vi "2024_06_02_sEQE.vi"() -> ()   [LabVIEW 2023]
uses:
  <vilib>/Utility/file.llb/Read From Spreadsheet File (DBL).vi
  <vilib>/gmath/NI_Gmath.lvlib
  <vilib>/Utility/file.llb/Write To Spreadsheet File (string).vi
  <vilib>/Utility/file.llb/Write To Spreadsheet File (DBL).vi
  Instrument Drivers/keithley_24xx/Keithley 24XX/Keithley 24XX.lvlib
  <vilib>/Analysis/NI_AALBase.lvlib
  E:/Old PC/desktop/Sensitive EQE Stuff/S-EQE (YJ)/Current Version/Thorlabs.MotionControl.Controls.dll
  <vilib>/Analysis/baseanly.llb/Mean (DBL).vi
  Files From Aram Lab/Labview VIs/EQE Newport/EQE Folder 2011/C/Program Files/National Instruments/LabVIEW 2017/instr.lib/Keithley 24XX/Public/Data/Read (Multiple Points).vi
  <vilib>/Analysis/1siggen.llb/Ramp Pattern by Samples.vi
  E:/Old PC/desktop/Sensitive EQE Stuff/S-EQE (YJ)/Current Version/Thorlabs.MotionControl.Benchtop.StepperMotorCLI.dll
panel:
  in  "Use Reference Detector":bool
  in  "Ref. Detector\nLockin Address":string="0:9"
  out "YJ@ AM1p5_1sun_photonflux_after interpolation":cluster{sgl[], "yi":dbl[]}(graph)
  out "70356_70316NS_473.txt":cluster{"all rows":dbl[], "all rows":dbl[]}(graph)={"all rows"=[0.0, 350.0, 355.0, 360.0, 365.0, 370.0, 375.0, 380.0, 385.0, 390.0, 395.0, 400.0, 405.0, 410.0, 415.0, 420.0, 425.0, 430.0, 435.0, 440.0, 445.0, 450.0, 455.0, 460.0, 465.0, 470.0, 475.0, 480.0, 485.0, 490.0, 495.0, 500.0, 505.0, 510.0, 515.0, 520.0, 525.0, 530.0, 535.0, 540.0, 545.0, 550.0, 555.0, 560.0, 565.0, 570.0, 575.0, 580.0, 585.0, 590.0, 595.0, 600.0, 605.0, 610.0, 615.0, 620.0, 625.0, 630.0, 635.0, 640.0, 645.0, 650.0, 655.0, 660.0, 665.0, 670.0, 675.0, 680.0, 685.0, 690.0, 695.0, 700.0, 705.0, 710.0, 715.0, 720.0, 725.0, 730.0, 735.0, 740.0, 745.0, 750.0, 755.0, 760.0, 765.0, 770.0, 775.0, 780.0, 785.0, 790.0, 795.0, 800.0, 805.0, 810.0, 815.0, 820.0, 825.0, 830.0, 835.0, 840.0, 845.0, 850.0, 855.0, 860.0, 865.0, 870.0, 875.0, 880.0, 885.0, 890.0, 895.0, 900.0, 905.0, 910.0, 915.0, 920.0, 925.0, 930.0, 935.0, 940.0, 945.0, 950.0, 955.0, 960.0, 965.0, 970.0, 975.0, 980.0, 985.0, 990.0, 995.0, 1000.0], "all rows"=[0.0, 0.000528, 0.000591, 0.00066, 0.000688, 0.000736, 0.000805, 0.000898, 0.000981, 0.001074, 0.001166, 0.001215, 0.001262, 0.001308, 0.001352, 0.001379, 0.001408, 0.001435, 0.001476, 0.001513, 0.00158, 0.001684, 0.001769, 0.001909, 0.002147, 0.002255, 0.002124, 0.002012, 0.001996, 0.001999, 0.00197, 0.001911, 0.001873, 0.001875, 0.00188, 0.001881, 0.001869, 0.001861, 0.001853, 0.00185, 0.001843, 0.001832, 0.001821, 0.001807, 0.001796, 0.001707, 0.001707, 0.001703, 0.001694, 0.001679, 0.00165, 0.001623, 0.001597, 0.001583, 0.001573, 0.001563, 0.00154, 0.001505, 0.001463, 0.00143, 0.001413, 0.001383, 0.001334, 0.001338, 0.001421, 0.001533, 0.001622, 0.00172, 0.00178, 0.001746, 0.001643, 0.001502, 0.001447, 0.001462, 0.001449, 0.001381, 0.001342, 0.001387, 0.001393, 0.001327, 0.001258, 0.001213, 0.001186, 0.001335, 0.001423, 0.001195, 0.000959, 0.000876, 0.000899, 0.000949, 0.00096, 0.000858, 0.000836, 0.000858, 0.001258, 0.002978, 0.00431, 0.003674, 0.002449, 0.001636, 0.001009, 0.000706, 0.000653, 0.000708, 0.000836, 0.001079, 0.001972, 0.003826, 0.004204, 0.003393, 0.003032, 0.00308, 0.002941, 0.002807, 0.003478, 0.003136, 0.001916, 0.001417, 0.001783, 0.002221, 0.002372, 0.002249, 0.001773, 0.001286, 0.001224, 0.001352, 0.002283, 0.002845, 0.002354, 0.002769, 0.002694, 0.001548]}
  out "YJ@ AM1p5_1sun_photonflux":cluster{"all rows":dbl[], "all rows":dbl[]}(graph)
  out "YJ@ KSC photodetector_Si_KSC.txt":cluster{"all rows":dbl[], "all rows":dbl[]}(graph)={"all rows"=[300.008, 319.964, 339.984, 359.993, 379.987, 399.968, 420.011, 440.038, 459.972, 479.966, 500.018, 519.975, 539.988, 559.982, 580.03, 599.981, 619.985, 639.966, 659.998, 680.005, 699.986, 720.017, 739.967, 759.964, 780.007, 800.019, 820.001, 840.026, 860.018, 879.977, 899.975, 920.013, 940.014, 959.979, 979.979, 1000.013, 1020.008, 1040.035, 1060.02, 1080.036, 1100.007, 1120.005, 1140.031, 1160.01, 1180.013, 1199.967, 1220.015, 1240.011, 1260.027, 1279.989, 1299.967, 1320.031, 1339.968, 1359.988, 1380.019, 1399.989, 1419.967, 1440.02, 1460.01, 1480.003, 1499.998, 1519.993, 1539.987, 1559.978, 1580.031, 1600.011, 1619.982, 1640.011, 1660.028, 1680.031, 1700.018, 1719.988, 1740.004, 1759.998, 1779.97, 1799.98], "all rows"=[22.44655, 29.69617, 32.2554, 33.72525, 44.35815, 59.92214, 69.4437, 73.3494, 73.77032, 72.54942, 69.11642, 66.67064, 64.65485, 63.26096, 62.09375, 61.11752, 61.04655, 61.202, 61.58933, 61.93196, 62.78305, 63.63964, 64.71529, 65.96744, 66.85927, 67.67915, 69.74085, 70.2863, 70.60146, 70.21348, 70.9341, 70.12613, 73.96691, 74.46643, 68.64919, 69.68867, 60.92799, 45.64385, 31.15813, 40.5953, 46.64548, 51.6218, 55.57125, 58.62437, 60.78791, 61.60885, 62.87273, 63.78579, 64.50757, 65.22985, 65.73163, 65.96526, 66.88447, 67.41929, 68.25897, 67.41081, 67.85151, 68.58292, 68.82948, 69.4892, 69.57728, 66.73863, 56.26826, 49.58999, 46.17923, 38.96613, 32.85697, 28.74497, 25.27677, 21.51941, 18.28548, 15.05667, 11.63632, 8.174946, 5.778172, 3.941114]}
  out "EQE data":dbl[](array[numeric])=[1.0630031270727235e-05, 2.224032414463779e-05, 3.860081064469949e-05, 5.693196442610228e-05, 7.885123421646286e-05, 0.00010409969342976093, 0.0001314805564755187, 0.00015761262171454783, 0.00018041038006170134, 0.0001994840969960363, 0.00021090229102895442, 0.00023735633466285739, 0.0002578215415721661, 0.00027707898011522546, 0.000293391194198478, 0.00031228191053828266, 0.0003277801105185816, 0.00033804597208761665, 0.0003483660325937561, 0.000366316440655734, 0.000385991499187727, 0.00042944053391323086, 0.000476573669238571, 0.0005114395273510304, 0.0005360105141446864, 0.0005518890213718105, 0.000554533572880275, 0.000545518555566591, 0.0005318038877618555, 0.0005248691938367492, 0.0005198235009739676, 0.0005139074960938296, 0.0005103600558364946, 0.0005099581034518405, 0.00051240772520516, 0.0005141352647575527, 0.0005160015247760515, 0.0005184268140636099, 0.0005215437161670573, 0.0005224495454948154, 0.0005239376083749391, 0.0005261934689407947, 0.0005275790524446975, 0.0005292676703269587, 3.684022279063007e-08, 3.001985497178216e-08, 3.011180213195135e-08, 6.376750400320879e-08, 6.389168834570928e-08, 6.305752891668185e-08]
  out "Applied Biases (V)":dbl[](array[numeric])
  out "Photonflux":dbl[](array[numeric])=[0.014905065, 0.017506614, 0.017369027, 0.018358634, 0.022533949, 0.017824447, 0.021478674, 0.020916015, 0.025070665, 0.025733941, 0.035944507, 0.037602476, 0.034673738, 0.041031376, 0.038050008, 0.042808518, 0.030334457, 0.043689466, 0.047907404, 0.05247181, 0.056603888, 0.05587127, 0.056733828, 0.057571786, 0.057155912, 0.062008993, 0.062646233, 0.061350661, 0.06412131, 0.065817672, 0.06231247, 0.06368507, 0.063682126, 0.06361276, 0.06390321, 0.066825496, 0.066029844, 0.06703682, 0.064570899, 0.067850258, 0.068313034, 0.069986046, 0.06657848, 0.069273794, 0.068116793, 0.068533433, 0.070266172, 0.07230634, 0.065238829, 0.068666398, 0.071397, 0.072684909, 0.0722573, 0.072904138, 0.073706888, 0.070706969, 0.070754315, 0.074050895, 0.074024843, 0.075784118, 0.071270366, 0.071316704, 0.074485562, 0.076240603, 0.076716567, 0.075993305, 0.076616551, 0.075958864, 0.065788756, 0.071271415, 0.072399581, 0.075140103, 0.075449669, 0.072589974, 0.057231812, 0.060699306, 0.066446604, 0.072195757, 0.072788353, 0.075094894, 0.074655186, 0.075408655, 0.016308308, 0.042329218, 0.072093563, 0.073580618, 0.073206001, 0.073358687, 0.069518471, 0.070099532, 0.06920471, 0.068468503, 0.06898524, 0.058849206, 0.057004485, 0.064503448, 0.061323463, 0.067565091, 0.068816583, 0.069280731, 0.061272947, 0.062962978, 0.068544733, 0.067204598, 0.067895507, 0.065414684, 0.066689918, 0.06740148, 0.066325028, 0.058730856, 0.053907082, 0.059644011, 0.045850113, 0.050064478, 0.055219293, 0.053054323, 0.032412728, 0.018917196, 0.035772012, 0.028065692, 0.011283836, 0.026279831, 0.032572479, 0.039208671, 0.049650887, 0.046388389, 0.047796935, 0.054673935, 0.058472923, 0.060332408, 0.059309566] format="%_6g"
  out "Gain (ohms, device)":dbl=1000.0
  out "Theta Device":dbl[](array[numeric])=[0.2700473581491309, 0.3151935612523878, 0.3840174824525091, 0.4343507017919065, 0.4985099952451927, 0.5521205217578055, 0.5932746185849422, 0.6229632673144792, 0.6603336996507065, 0.7021736365126859, 0.730245402674861, 0.7555351998358408, 0.7662251733370439, 0.7732410218978927, 0.7868403454893664, 0.8079871608349878, 0.833604606370508, 0.8512186270266459, 0.8571435014368394, 0.849056818576912, 0.8230805736611391, 0.797472299831973, 0.7949251497551506, 0.8229193465162005, 0.8544820820870439, 0.8945387107767107, 0.9101509858937846, 0.9180726508270242, 0.9138050297047764, 0.9170227233725305, 0.9185973975743922, 0.9127798480771039, 0.9020006840177286, 0.9085453202656186, 0.9004761874895579, 0.9060028541494218, 0.9048110423655178, 0.9040744374822528, 0.9048831165145835, 0.9054391223829343, 0.9038549251113345, 0.9099900965130696, 0.9091406237134004, 0.905658502401197, 0.9696722358529832, 0.9234869853808101, 0.8983673358190203, 0.6879877400938528, 0.6622097148496295, 0.6684745327767915]
  out "Calib Ref Current":dbl=1.455414177111583e-07
  out "Calib Photodet Current":dbl=1.1887647122469343e-06
  out "Calib detector EQE":dbl=0.7476
  out "Gain (ohms, ref)":dbl=1000.0
  out "Reference Current (A)":dbl[](array[numeric])=[0.001, 0.001, 0.001, 0.001, 0.001, 0.001, 0.001, 0.001, 0.001, 0.001, 0.001, 0.001, 0.001, 0.001, 0.001, 0.001, 0.001, 0.001, 0.001, 0.001, 0.001, 0.001, 0.001, 0.001, 0.001, 0.001, 0.001, 0.001, 0.001, 0.001, 0.001, 0.001, 0.001, 0.001, 0.001, 0.001, 0.001, 0.001, 0.001, 0.001, 0.001, 0.001, 0.001, 0.001, 0.001, 0.001, 0.001, 0.001, 0.001, 0.001]
  out "DC current (A)":dbl[](array[numeric])
  out "Device Current (A)":dbl[](array[numeric])=[3.506971664575117e-07, 7.419031190448685e-07, 1.3019656857999596e-06, 2.0716400561544406e-06, 3.0789055653533614e-06, 4.3415860564758075e-06, 5.833565646397709e-06, 7.606853812813335e-06, 9.409785273244745e-06, 1.1181556134893594e-05, 1.2640922706358269e-05, 1.4790296262148529e-05, 1.66779361860275e-05, 1.8581800630899686e-05, 2.037263692081463e-05, 2.1989850169184038e-05, 2.3400802905737088e-05, 2.4463332489649517e-05, 2.5549857791294584e-05, 2.6907472308324217e-05, 2.8393439889071035e-05, 3.1634879861557116e-05, 3.515617725054383e-05, 3.757203217284588e-05, 3.92134448854471e-05, 4.020658347574139e-05, 4.0227861162201044e-05, 3.9106902201208186e-05, 3.7668493858212035e-05, 3.6727997932696076e-05, 3.592994135283064e-05, 3.520567678187613e-05, 3.464992685110582e-05, 3.4310153885847094e-05, 3.416126068610294e-05, 3.4017503626001664e-05, 3.388111502655533e-05, 3.3779271471066726e-05, 3.3719894421586654e-05, 3.359634598967278e-05, 3.350940388445748e-05, 3.347026266189864e-05, 3.3374604444484423e-05, 3.3327354406248036e-05, 2.309060591324272e-09, 1.872836698407875e-09, 1.8698073076001774e-09, 3.944055898210585e-09, 3.936105226456829e-09, 3.869288620508274e-09]
  out "Wavelength range":sgl[](array[numeric])=[350.0, 355.0, 360.0, 365.0, 370.0, 375.0, 380.0, 385.0, 390.0, 395.0, 400.0, 405.0, 410.0, 415.0, 420.0, 425.0, 430.0, 435.0, 440.0, 445.0, 450.0, 455.0, 460.0, 465.0, 470.0, 475.0, 480.0, 485.0, 490.0, 495.0, 500.0, 505.0, 510.0, 515.0, 520.0, 525.0, 530.0, 535.0, 540.0, 545.0, 550.0, 555.0, 560.0, 565.0, 570.0, 575.0, 580.0, 585.0, 590.0, 595.0, 600.0, 605.0, 610.0, 615.0, 620.0, 625.0, 630.0, 635.0, 640.0, 645.0, 650.0, 655.0, 660.0, 665.0, 670.0, 675.0, 680.0, 685.0, 690.0, 695.0, 700.0, 705.0, 710.0, 715.0, 720.0, 725.0, 730.0, 735.0, 740.0, 745.0, 750.0, 755.0, 760.0, 765.0, 770.0, 775.0, 780.0, 785.0, 790.0, 795.0, 800.0, 805.0, 810.0, 815.0, 820.0, 825.0, 830.0, 835.0, 840.0, 845.0, 850.0, 855.0, 860.0, 865.0, 870.0, 875.0, 880.0, 885.0, 890.0, 895.0, 900.0, 905.0, 910.0, 915.0, 920.0, 925.0, 930.0, 935.0, 940.0, 945.0, 950.0, 955.0, 960.0, 965.0, 970.0, 975.0, 980.0, 985.0, 990.0, 995.0, 1000.0, 1005.0, 1010.0, 1015.0, 1020.0, 1025.0, 1030.0, 1035.0, 1040.0, 1045.0, 1050.0]
  in  "Tab Control":T1(tab)
  out "Auto Scale":string="Successful"
  out "Lockin status":bool
  out "Position of filter 1":dbl=360.0
  in  "Set as filter 1":bool
  out "Current degree":dbl=60.0
  out "Rotator status":bool
  in  "Anticlockwise":bool
  in  "clockwise":bool
  out "Mono status":bool
  out "Keithley status":bool
  in  "Initial devices":bool caption="To be initialized"
  in  "Start EXP":bool
  in  "Use Keithley for Bias?":bool
  in  "stop 3":bool caption="Be patient with this function"
  out "Current Wavelength":dbl=600.0 min=350.0 max=1100.0 step=1.0 format="%#.1f"
  out "Integrated Photocurrent (mA/cm2):":dbl format="%#_4f"
  in  "FileIO":enum32{"Take Calibration", "Take Measurement"}(tab)
  in  "Load Calibration Reference file":path=path "E:/Old PC/desktop/Sensitive EQE Stuff/S-EQE (YJ)/Calibration files (YJ)/JPJ New/KSC Combined Detector JPJ.txt"
  in  "70356_70316NS_473.txt":path=path "C:/Users/Admin/Desktop/Sensitive EQE Stuff/S-EQE (YJ)/Calibration files (YJ)/Si_Calibtation 19022019"
  out "70356_70316NS_473 File":cluster{sgl[], "yi":dbl[]}(graph)={[350.0, 355.0, 360.0, 365.0, 370.0, 375.0, 380.0, 385.0, 390.0, 395.0, 400.0, 405.0, 410.0, 415.0, 420.0, 425.0, 430.0, 435.0, 440.0, 445.0, 450.0, 455.0, 460.0, 465.0, 470.0, 475.0, 480.0, 485.0, 490.0, 495.0, 500.0, 505.0, 510.0, 515.0, 520.0, 525.0, 530.0, 535.0, 540.0, 545.0, 550.0, 555.0, 560.0, 565.0, 570.0, 575.0, 580.0, 585.0, 590.0, 595.0, 600.0, 605.0, 610.0, 615.0, 620.0, 625.0, 630.0, 635.0, 640.0, 645.0, 650.0, 655.0, 660.0, 665.0, 670.0, 675.0, 680.0, 685.0, 690.0, 695.0, 700.0, 705.0, 710.0, 715.0, 720.0, 725.0, 730.0, 735.0, 740.0, 745.0, 750.0, 755.0, 760.0, 765.0, 770.0, 775.0, 780.0, 785.0, 790.0, 795.0, 800.0, 805.0, 810.0, 815.0, 820.0, 825.0, 830.0, 835.0, 840.0, 845.0, 850.0, 855.0, 860.0, 865.0, 870.0, 875.0, 880.0, 885.0, 890.0, 895.0, 900.0, 905.0, 910.0, 915.0, 920.0, 925.0, 930.0, 935.0, 940.0, 945.0, 950.0, 955.0, 960.0, 965.0, 970.0, 975.0, 980.0, 985.0, 990.0, 995.0, 1000.0, 1005.0, 1010.0, 1015.0, 1020.0, 1025.0, 1030.0, 1035.0, 1040.0, 1045.0, 1050.0], "yi"=[32.991169783597385, 33.35846699985007, 33.728972631789546, 36.38799533860158, 39.04701804541362, 41.70604075222566, 44.368276213402716, 48.26297367599218, 52.15767113858164, 56.052368601171096, 59.937341812103966, 62.31262495335029, 64.68790809459661, 67.06319123584294, 69.43847437708925, 70.41666336445799, 71.39177196784341, 72.36688057122885, 73.34198917461427, 73.45417601284238, 73.55975442159125, 73.66533283034012, 73.76861022706812, 73.46329363208963, 73.15797703711112, 72.85266044213263, 72.54359903451027, 71.68757469778576, 70.83155036106125, 69.97552602433672, 69.11950168761221, 68.50586350553691, 67.89310106629253, 67.28033862704817, 66.66812189926549, 66.16450175236098, 65.66088160545645, 65.15726145855194, 64.65401341502451, 64.30543634190258, 63.95685926878063, 63.608282195658695, 63.259912026137265, 62.96880817537909, 62.677704324620905, 62.38660047386273, 62.095496623104545, 61.850561032028466, 61.60590412260037, 61.36124721317227, 61.1174525919816, 61.09971363977205, 61.081974687562486, 61.06423573535293, 61.046666698363445, 61.0855661528452, 61.12446560732696, 61.16336506180872, 61.20265740914537, 61.29933522464057, 61.39601304013578, 61.49269085563099, 61.58936425101214, 61.67499178137651, 61.76061931174089, 61.84624684210526, 61.931874372469636, 62.144721851258694, 62.357696677343476, 62.57067150342826, 62.783648685038195, 62.99746477010633, 63.21128085517448, 63.425096940242625, 63.63891302531077, 63.908309872180446, 64.17789633834586, 64.44748280451128, 64.71735635745361, 65.03044082012302, 65.34352528279241, 65.65660974546181, 65.96904185002245, 66.19152101980741, 66.41400018959237, 66.63647935937733, 66.8589585291623, 67.06383030581651, 67.26867739756146, 67.47352448930641, 67.67837158105138, 68.19307892102893, 68.70896822139926, 69.2248575217696, 69.74074682213993, 69.87701502122347, 70.01320728089887, 70.14939954057428, 70.28559180024969, 70.36471165666266, 70.4435331852741, 70.52235471388555, 70.601176242497, 70.50461565108473, 70.4074214028759, 70.31022715466707, 70.21430879587959, 70.39448181318133, 70.57465483048306, 70.75482784778478, 70.93309195278971, 70.73148251072962, 70.52987306866953, 70.32826362660944, 70.12665418454937, 71.08378061046947, 72.04392760311985, 73.0040745957702, 73.96422158842057, 74.09165864613072, 74.21675756924618, 74.34185649236163, 74.460321898, 73.00601189800001, 71.551701898, 70.09739189800001, 68.65027960167716, 68.90970857242688, 69.1691375431766, 69.42856651392633, 69.68799548467605, 67.50364818654668, 65.31293050712678, 63.12221282770695, 60.93149514828712, 57.11821185649378, 53.302328299296015, 49.48644474209825, 45.670561184900485, 42.04507092569435, 38.42092281461098]}
  out "Lamp Reference Photodetector Current":cluster{"Wavelength range":sgl[], dbl[]}(graph)={"Wavelength range"=[350.0, 355.0, 360.0, 365.0, 370.0, 375.0, 380.0, 385.0, 390.0, 395.0, 400.0, 405.0, 410.0, 415.0, 420.0, 425.0, 430.0, 435.0, 440.0, 445.0, 450.0, 455.0, 460.0, 465.0, 470.0, 475.0, 480.0, 485.0, 490.0, 495.0, 500.0, 505.0, 510.0, 515.0, 520.0, 525.0, 530.0, 535.0, 540.0, 545.0, 550.0, 555.0, 560.0, 565.0, 570.0, 575.0, 580.0, 585.0, 590.0, 595.0, 600.0, 605.0, 610.0, 615.0, 620.0, 625.0, 630.0, 635.0, 640.0, 645.0, 650.0, 655.0, 660.0, 665.0, 670.0, 675.0, 680.0, 685.0, 690.0, 695.0, 700.0, 705.0, 710.0, 715.0, 720.0, 725.0, 730.0, 735.0, 740.0, 745.0, 750.0, 755.0, 760.0, 765.0, 770.0, 775.0, 780.0, 785.0, 790.0, 795.0, 800.0, 805.0, 810.0, 815.0, 820.0, 825.0, 830.0, 835.0, 840.0, 845.0, 850.0, 855.0, 860.0, 865.0, 870.0, 875.0, 880.0, 885.0, 890.0, 895.0, 900.0, 905.0, 910.0, 915.0, 920.0, 925.0, 930.0, 935.0, 940.0, 945.0, 950.0, 955.0, 960.0, 965.0, 970.0, 975.0, 980.0, 985.0, 990.0, 995.0, 1000.0, 1005.0, 1010.0, 1015.0, 1020.0, 1025.0, 1030.0, 1035.0, 1040.0, 1045.0, 1050.0], [0.001, 0.001, 0.001, 0.001, 0.001, 0.001, 0.001, 0.001, 0.001, 0.001, 0.001, 0.001, 0.001, 0.001, 0.001, 0.001, 0.001, 0.001, 0.001, 0.001, 0.001, 0.001, 0.001, 0.001, 0.001, 0.001, 0.001, 0.001, 0.001, 0.001, 0.001, 0.001, 0.001, 0.001, 0.001, 0.001, 0.001, 0.001, 0.001, 0.001, 0.001, 0.001, 0.001, 0.001, 0.001, 0.001, 0.001, 0.001, 0.001, 0.001]}
  out "Device Current":cluster{"Wavelength range":sgl[], dbl[]}(graph)={"Wavelength range"=[350.0, 355.0, 360.0, 365.0, 370.0, 375.0, 380.0, 385.0, 390.0, 395.0, 400.0, 405.0, 410.0, 415.0, 420.0, 425.0, 430.0, 435.0, 440.0, 445.0, 450.0, 455.0, 460.0, 465.0, 470.0, 475.0, 480.0, 485.0, 490.0, 495.0, 500.0, 505.0, 510.0, 515.0, 520.0, 525.0, 530.0, 535.0, 540.0, 545.0, 550.0, 555.0, 560.0, 565.0, 570.0, 575.0, 580.0, 585.0, 590.0, 595.0, 600.0, 605.0, 610.0, 615.0, 620.0, 625.0, 630.0, 635.0, 640.0, 645.0, 650.0, 655.0, 660.0, 665.0, 670.0, 675.0, 680.0, 685.0, 690.0, 695.0, 700.0, 705.0, 710.0, 715.0, 720.0, 725.0, 730.0, 735.0, 740.0, 745.0, 750.0, 755.0, 760.0, 765.0, 770.0, 775.0, 780.0, 785.0, 790.0, 795.0, 800.0, 805.0, 810.0, 815.0, 820.0, 825.0, 830.0, 835.0, 840.0, 845.0, 850.0, 855.0, 860.0, 865.0, 870.0, 875.0, 880.0, 885.0, 890.0, 895.0, 900.0, 905.0, 910.0, 915.0, 920.0, 925.0, 930.0, 935.0, 940.0, 945.0, 950.0, 955.0, 960.0, 965.0, 970.0, 975.0, 980.0, 985.0, 990.0, 995.0, 1000.0, 1005.0, 1010.0, 1015.0, 1020.0, 1025.0, 1030.0, 1035.0, 1040.0, 1045.0, 1050.0], [3.506971664575117e-07, 7.419031190448685e-07, 1.3019656857999596e-06, 2.0716400561544406e-06, 3.0789055653533614e-06, 4.3415860564758075e-06, 5.833565646397709e-06, 7.606853812813335e-06, 9.409785273244745e-06, 1.1181556134893594e-05, 1.2640922706358269e-05, 1.4790296262148529e-05, 1.66779361860275e-05, 1.8581800630899686e-05, 2.037263692081463e-05, 2.1989850169184038e-05, 2.3400802905737088e-05, 2.4463332489649517e-05, 2.5549857791294584e-05, 2.6907472308324217e-05, 2.8393439889071035e-05, 3.1634879861557116e-05, 3.515617725054383e-05, 3.757203217284588e-05, 3.92134448854471e-05, 4.020658347574139e-05, 4.0227861162201044e-05, 3.9106902201208186e-05, 3.7668493858212035e-05, 3.6727997932696076e-05, 3.592994135283064e-05, 3.520567678187613e-05, 3.464992685110582e-05, 3.4310153885847094e-05, 3.416126068610294e-05, 3.4017503626001664e-05, 3.388111502655533e-05, 3.3779271471066726e-05, 3.3719894421586654e-05, 3.359634598967278e-05, 3.350940388445748e-05, 3.347026266189864e-05, 3.3374604444484423e-05, 3.3327354406248036e-05, 2.309060591324272e-09, 1.872836698407875e-09, 1.8698073076001774e-09, 3.944055898210585e-09, 3.936105226456829e-09, 3.869288620508274e-09]}
  in  "Step size (nm)":sgl=5.0 min=1 step=0.1
  in  "End Wavelength (nm)":sgl=1050.0 min=250 max=1350 step=0.1
  in  "Start Wavelength (nm)":sgl=350.0 min=250 max=1200 step=0.1
  in  "Bias (V)":dbl min=-30.0 max=10.0
  out "EQE":cluster{"Wavelength range":sgl[], dbl[]}(graph)={"Wavelength range"=[350.0, 355.0, 360.0, 365.0, 370.0, 375.0, 380.0, 385.0, 390.0, 395.0, 400.0, 405.0, 410.0, 415.0, 420.0, 425.0, 430.0, 435.0, 440.0, 445.0, 450.0, 455.0, 460.0, 465.0, 470.0, 475.0, 480.0, 485.0, 490.0, 495.0, 500.0, 505.0, 510.0, 515.0, 520.0, 525.0, 530.0, 535.0, 540.0, 545.0, 550.0, 555.0, 560.0, 565.0, 570.0, 575.0, 580.0, 585.0, 590.0, 595.0, 600.0, 605.0, 610.0, 615.0, 620.0, 625.0, 630.0, 635.0, 640.0, 645.0, 650.0, 655.0, 660.0, 665.0, 670.0, 675.0, 680.0, 685.0, 690.0, 695.0, 700.0, 705.0, 710.0, 715.0, 720.0, 725.0, 730.0, 735.0, 740.0, 745.0, 750.0, 755.0, 760.0, 765.0, 770.0, 775.0, 780.0, 785.0, 790.0, 795.0, 800.0, 805.0, 810.0, 815.0, 820.0, 825.0, 830.0, 835.0, 840.0, 845.0, 850.0, 855.0, 860.0, 865.0, 870.0, 875.0, 880.0, 885.0, 890.0, 895.0, 900.0, 905.0, 910.0, 915.0, 920.0, 925.0, 930.0, 935.0, 940.0, 945.0, 950.0, 955.0, 960.0, 965.0, 970.0, 975.0, 980.0, 985.0, 990.0, 995.0, 1000.0, 1005.0, 1010.0, 1015.0, 1020.0, 1025.0, 1030.0, 1035.0, 1040.0, 1045.0, 1050.0], [1.0630031270727235e-05, 2.224032414463779e-05, 3.860081064469949e-05, 5.693196442610228e-05, 7.885123421646286e-05, 0.00010409969342976093, 0.0001314805564755187, 0.00015761262171454783, 0.00018041038006170134, 0.0001994840969960363, 0.00021090229102895442, 0.00023735633466285739, 0.0002578215415721661, 0.00027707898011522546, 0.000293391194198478, 0.00031228191053828266, 0.0003277801105185816, 0.00033804597208761665, 0.0003483660325937561, 0.000366316440655734, 0.000385991499187727, 0.00042944053391323086, 0.000476573669238571, 0.0005114395273510304, 0.0005360105141446864, 0.0005518890213718105, 0.000554533572880275, 0.000545518555566591, 0.0005318038877618555, 0.0005248691938367492, 0.0005198235009739676, 0.0005139074960938296, 0.0005103600558364946, 0.0005099581034518405, 0.00051240772520516, 0.0005141352647575527, 0.0005160015247760515, 0.0005184268140636099, 0.0005215437161670573, 0.0005224495454948154, 0.0005239376083749391, 0.0005261934689407947, 0.0005275790524446975, 0.0005292676703269587, 3.684022279063007e-08, 3.001985497178216e-08, 3.011180213195135e-08, 6.376750400320879e-08, 6.389168834570928e-08, 6.305752891668185e-08]}
  out "EQE (log scale)":cluster{"Wavelength range":sgl[], dbl[]}(graph)={"Wavelength range"=[350.0, 355.0, 360.0, 365.0, 370.0, 375.0, 380.0, 385.0, 390.0, 395.0, 400.0, 405.0, 410.0, 415.0, 420.0, 425.0, 430.0, 435.0, 440.0, 445.0, 450.0, 455.0, 460.0, 465.0, 470.0, 475.0, 480.0, 485.0, 490.0, 495.0, 500.0, 505.0, 510.0, 515.0, 520.0, 525.0, 530.0, 535.0, 540.0, 545.0, 550.0, 555.0, 560.0, 565.0, 570.0, 575.0, 580.0, 585.0, 590.0, 595.0, 600.0, 605.0, 610.0, 615.0, 620.0, 625.0, 630.0, 635.0, 640.0, 645.0, 650.0, 655.0, 660.0, 665.0, 670.0, 675.0, 680.0, 685.0, 690.0, 695.0, 700.0, 705.0, 710.0, 715.0, 720.0, 725.0, 730.0, 735.0, 740.0, 745.0, 750.0, 755.0, 760.0, 765.0, 770.0, 775.0, 780.0, 785.0, 790.0, 795.0, 800.0, 805.0, 810.0, 815.0, 820.0, 825.0, 830.0, 835.0, 840.0, 845.0, 850.0, 855.0, 860.0, 865.0, 870.0, 875.0, 880.0, 885.0, 890.0, 895.0, 900.0, 905.0, 910.0, 915.0, 920.0, 925.0, 930.0, 935.0, 940.0, 945.0, 950.0, 955.0, 960.0, 965.0, 970.0, 975.0, 980.0, 985.0, 990.0, 995.0, 1000.0, 1005.0, 1010.0, 1015.0, 1020.0, 1025.0, 1030.0, 1035.0, 1040.0, 1045.0, 1050.0], [1.0630031270727235e-05, 2.224032414463779e-05, 3.860081064469949e-05, 5.693196442610228e-05, 7.885123421646286e-05, 0.00010409969342976093, 0.0001314805564755187, 0.00015761262171454783, 0.00018041038006170134, 0.0001994840969960363, 0.00021090229102895442, 0.00023735633466285739, 0.0002578215415721661, 0.00027707898011522546, 0.000293391194198478, 0.00031228191053828266, 0.0003277801105185816, 0.00033804597208761665, 0.0003483660325937561, 0.000366316440655734, 0.000385991499187727, 0.00042944053391323086, 0.000476573669238571, 0.0005114395273510304, 0.0005360105141446864, 0.0005518890213718105, 0.000554533572880275, 0.000545518555566591, 0.0005318038877618555, 0.0005248691938367492, 0.0005198235009739676, 0.0005139074960938296, 0.0005103600558364946, 0.0005099581034518405, 0.00051240772520516, 0.0005141352647575527, 0.0005160015247760515, 0.0005184268140636099, 0.0005215437161670573, 0.0005224495454948154, 0.0005239376083749391, 0.0005261934689407947, 0.0005275790524446975, 0.0005292676703269587, 3.684022279063007e-08, 3.001985497178216e-08, 3.011180213195135e-08, 6.376750400320879e-08, 6.389168834570928e-08, 6.305752891668185e-08]}
  in  "Pause Request":bool
  out "Paused":bool
  in  "Keithley 2400 address":refnum<visa-resource-name>="GPIB0::24::INSTR"
  in  "AM1p5_1sun_photoflux":path=path "E:/Old PC/desktop/Sensitive EQE Stuff/S-EQE (YJ)/Calibration files (YJ)/AM1p5_1sun_photonflux.xls"
  in  "Step":string(combo)="60"
  out "Delay (s)":sgl=1.5 format="%#.2f"
  in  "lockin":T2={"Lock-in VISA address"="GPIB0::8::INSTR", "Integration (ms) "=3000, "data storage rate (Hz)"=enum."16"}
  out "GPIB address":string="0:8"
  in  "Autogain":bool
  in  "stop":bool
  out "Current Filter":dbl=5.0
  in  "Autoscale Starts":dbl=350.0
  in  "Auto Gain Point Separation":i32=1
  in  "Average Method":bool=TRUE
  in  "Delay-2 (s)":dbl=5.0
  in  "MC Config File (19523)":path=path "E:/Old PC/desktop/MSH-300/MSH-300/Configurations/config/19523/LOT_MSH-300_SN19523 new (1).xml"
  out "Current wavelength test (nm)":dbl=550.0 format="%#.1f"
  in  "Goto wavelength":bool
  in  "Wavelength (nm)":sgl=550.0 min=250 max=1350 step=0.1 format="%.1f"
  in  "Skip reset after\nmeasurement":bool
  in  "Save File (Prompt if blank)":path
  in  "Voltage Profile":path=path "C:/Labview VIs/Voltage Profiles/ETH_1.xls"
  in  "Load Voltage Profile?":bool
  in  "Lock-In IV curve calb tab":enum32{"Calibrate", "Scan"}(tab)
  in  "Load Calibration Reference file":path=path "C:/Labview VIs/Photodiode Calibration Files/70356_70316NS_473.txt"
  in  "Calibration Value":dbl=11.66 min=0.0
  in  "Use Reference Detector?":bool=TRUE
  in  "Lockin Parameters":T3={"Device Lockin Address"="1:8", "Ref. Lockin Address"="1:9", "Wait (ms)"=500.0, "Integration (ms) "=2000, "data storage rate (Hz)"=enum."32"}
  in  "Monochromator Controls":T4={"Wavelength (nm)"=550.0, "Shutter"=enum."Open"} {"Wavelength (nm)" min=0 max=1400 step=0.1}
  out "EQE(V)":cluster{dbl[], dbl[]}(graph)={[0.0], [5.834199398071779]}
  out "Reference Lockin Current":cluster{"Wavelengths":dbl[], dbl[]}(graph)={"Wavelengths"=[0.0], [1.455414177111583e-07]}
  out "Device Lockin Current":cluster{dbl[], dbl[]}(graph)={[0.0], [1.1887647122469343e-06]}
  out "Device DC current":cluster{dbl[], dbl[]}(graph)={[0.0], [1.0150755315407879e-06]}
  in  "Bias Parameters":T5={"VISA resource name"="GPIB0::24::INSTR", "Start Bias (V)"=1.0, "End Bias (V) "=-10.0, "Number of points minus 1"=50, "Compliance (A)"=0.05} {"Number of points minus 1" min=0}
  in  "stop 2":bool
  in  "BenchtopStepperControl":refnum<k24>(container)
  out "BenchtopStepperMotor":refnum<k24>
  # "YJ@Select the measurement rage"
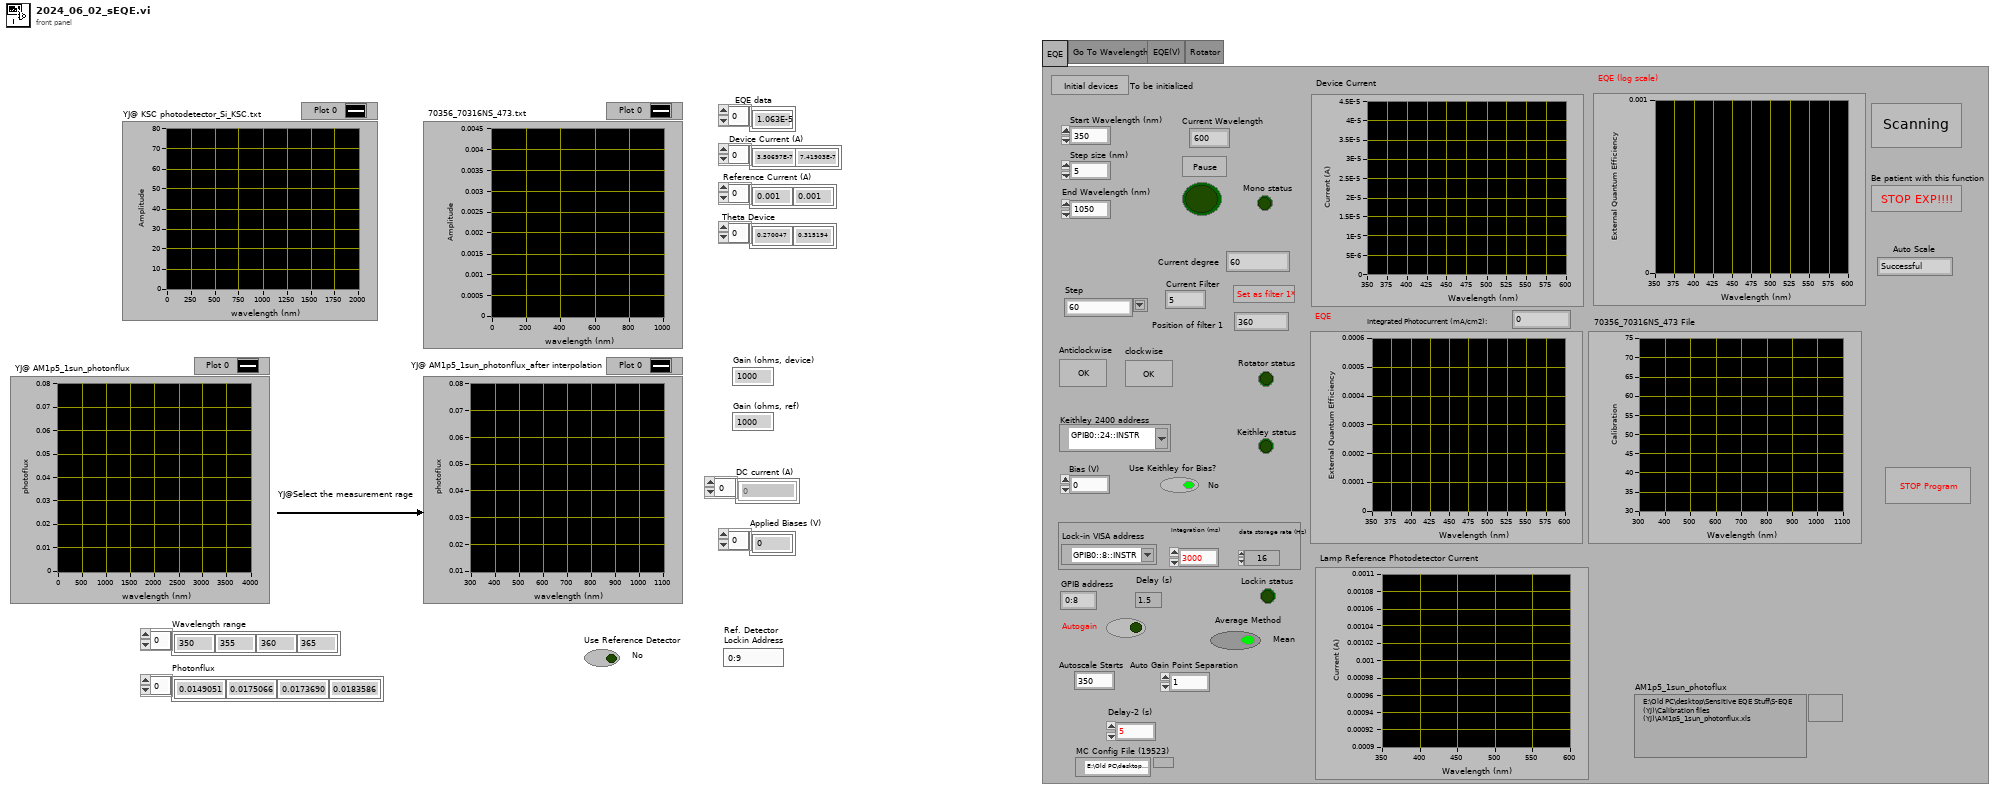
[diagram p1: front panel]
types:
  T1 = enum32{"EQE", "Go To Wavelength", "EQE(V)", "Rotator"}
  T2 = cluster{"Lock-in VISA address":refnum<visa-resource-name>, "Integration (ms) ":u32, "data storage rate (Hz)":enum16{".0625", ".125", ".25", ".5", "1", "2", "4", "8", "16", "32", "64", "128", "256", "512"}}
  T3 = cluster{"Device Lockin Address":string, "Ref. Lockin Address":string, "Wait (ms)":dbl, "Integration (ms) ":u32, "data storage rate (Hz)":enum16{".0625", ".125", ".25", ".5", "1", "2", "4", "8", "16", "32", "64", "128", "256", "512"}}
  T4 = cluster{"Wavelength (nm)":sgl, "Shutter":enum16{"Open", "Closed"}}
  T5 = cluster{"VISA resource name":refnum<visa-resource-name>, "Start Bias (V)":dbl, "End Bias (V) ":dbl, "Number of points minus 1":i16, "Compliance (A)":dbl}
  T6 = enum8{"Enabled", "Disabled", "Disabled and Grayed Out"}
  T7 = enum16{".0625", ".125", ".25", ".5", "1", "2", "4", "8", "16", "32", "64", "128", "256", "512"}
  T8 = cluster{"error":bool, "code":i32, "source":string}
  T9 = cluster{"Applied Biases (V)":dbl[], "DC current (A)":dbl[]}
  T10 = cluster{"Applied Biases (V)":dbl[], "Device Current (A)":dbl[]}
  T11 = cluster{"Applied Biases (V)":dbl[], "Reference Current (A)":dbl[]}
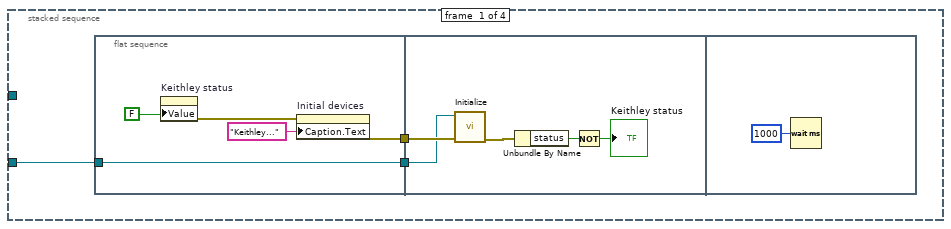
[diagram p6: hidden frame]
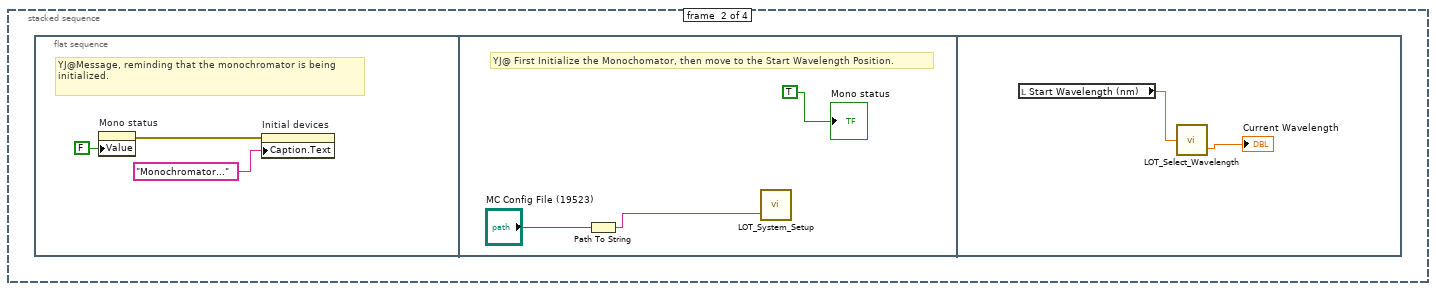
[diagram p7: hidden frame]
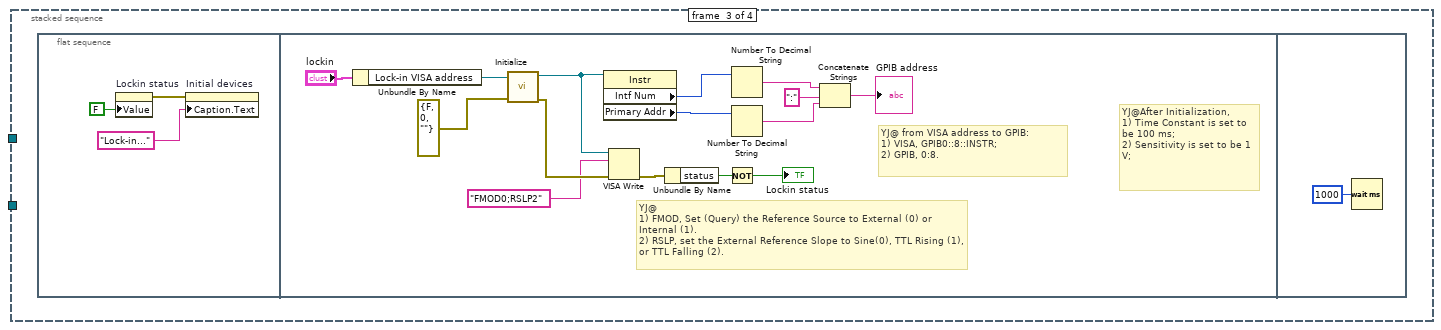
[diagram p8: hidden frame]
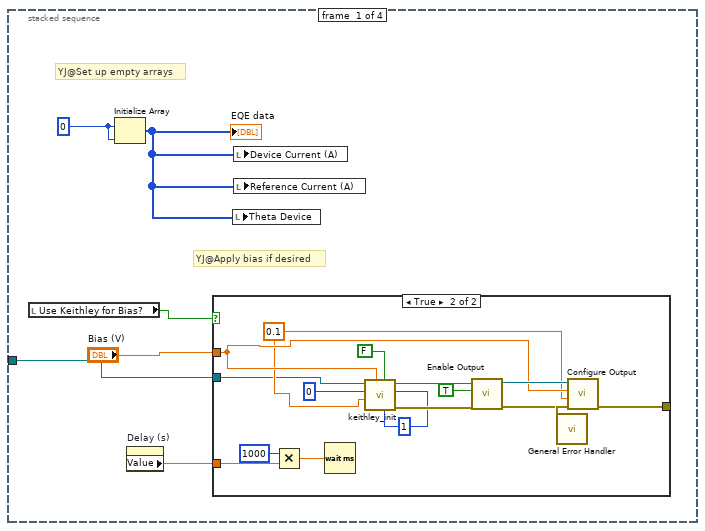
[diagram p10: hidden frame]
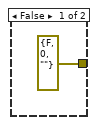
[diagram p11: hidden frame]
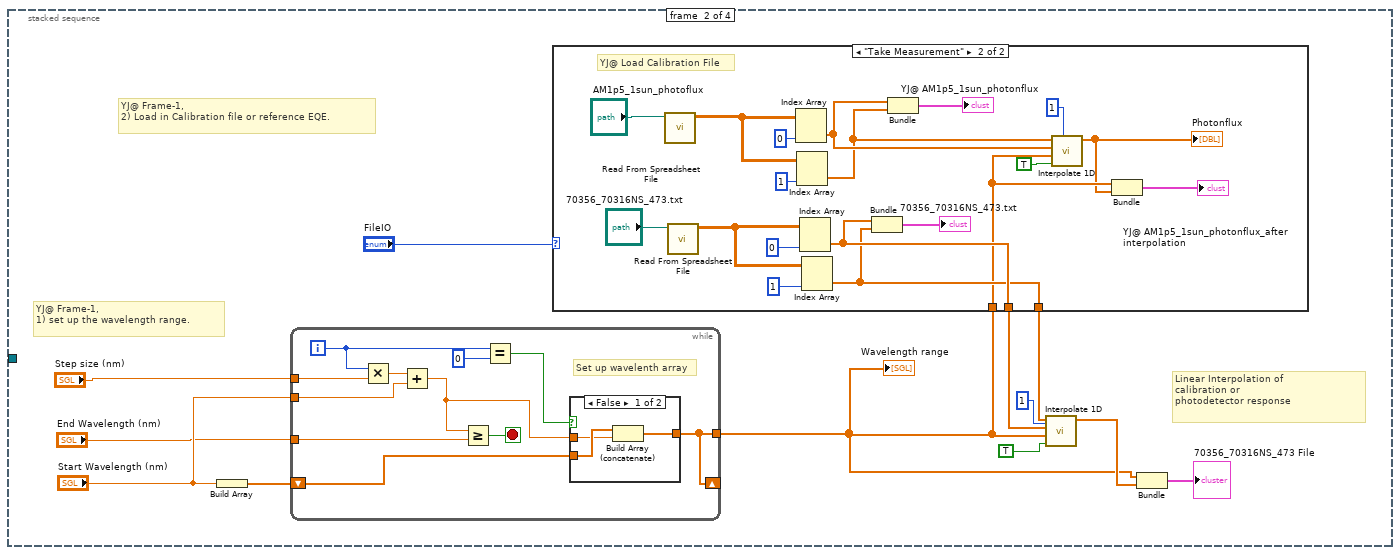
[diagram p12: hidden frame]
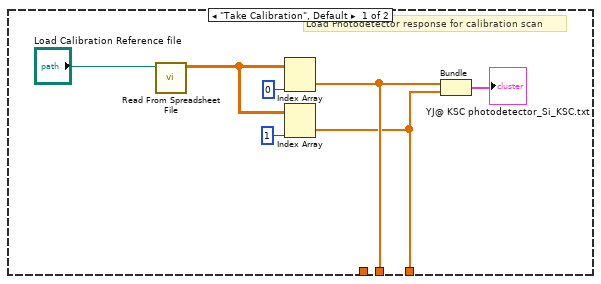
[diagram p14: hidden frame]
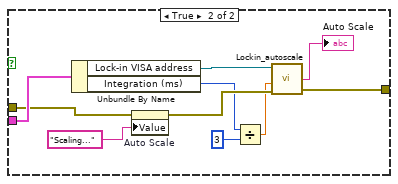
[diagram p15: hidden frame]
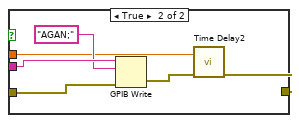
[diagram p17: hidden frame]
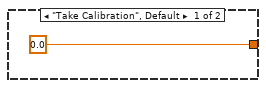
[diagram p18: hidden frame]
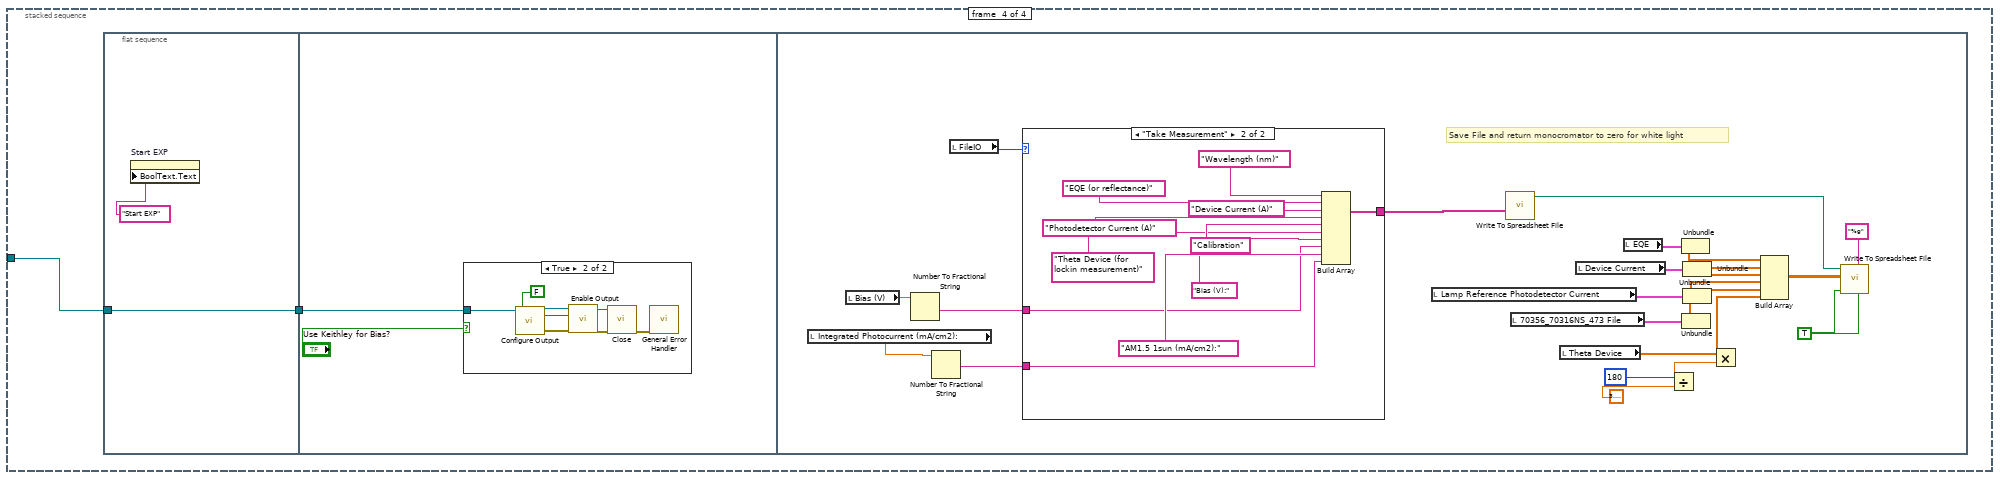
[diagram p19: hidden frame]
diagram:
  w2 = FALSE ("Lockin status")
  # "YJ@\n1)Delay time is one half of the integration;\n2)Be careful for the unit conversion, Integration being ms, and delay being second."
  n1 = property on="Rotator status" class="Bool (strict)"("Value"=w2) -> ()  [unwired: 2 in, 2 out]
  n2 = property on="Mono status" class="Bool (strict)"("Value"=w2) -> ()  [unwired: 2 in, 2 out]
  n3 = property on="Keithley status" class="Bool (strict)"("Value"=w2) -> ()  [unwired: 2 in, 2 out]
  n4 = property on="Lockin status" class="Bool (strict)"("Value"=w2) -> (error out=w3:errorcluster)  [unwired: 2 in, 1 out]
  n5 = property on="Position of filter 1" class="DigNum (strict)"("Value"=360.0 ("Position of filter 1")) -> ()  [unwired: 2 in, 2 out]
  n6 = property on="Start EXP" class="Bool"(error in=w3, "BoolText.Text"="Start EXP" ("Boolean Text.Text")) -> (error out=w5:errorcluster)  [unwired: 1 in, 1 out]
  n7 = property on="Initial devices" class="Bool"(error in=w5, "Caption.Text"="To be initialized") -> (error out=w6:errorcluster)  [unwired: 1 in, 1 out]
  n8 = while "Level-1, while loop, controlling the whole S-EQE program." {
    tunnel: w6 -> [w8]
    stop <- "stop" stop-if-true
    # "YJ@four tabs:\n1, EQE;\n2, Go To Wavelength;\n3, EQE (V);\n4, Rotator;"
    n9 = property on="lockin" class="Clust (strict)"(error in=w8) -> ("Value"=w10:T2)  [unwired: 1 in, 2 out]
    n10 = Unbundle By Name(w10) -> ("Integration (ms)"=w11:u32)
    n11 = Wait (ms)(milliseconds to wait=u32 20) -> ()  [unwired: 1 out]
    n12 = Divide(x=w11, y=u32 2000) -> (x/y=→"Delay (s)":dbl)
    n13 = case "Level-2, case structure, controlled by Tab Control, choosing specific pages." shown="\"EQE\", Default" "Tab Control" {
      tunnel: "Keithley 2400 address" -> [w31 _ _]
      frame "EQE", Default {
        n14 = case "Level-3, case structure, controlled by OK buttong, determine whether to initiate the units or not." shown="True" "Initial devices" {
          tunnel: w31 -> [_ w55]
          tunnel: "BenchtopStepperControl" -> [_ w54]
          frame False {
          }
          frame True {
            # "YJ@A sequence of Initialization:\nFrame-0, Keithley;\nFrame-1,Mono-chromator;\nFrame-2, Lock-in;\nFrame-3, Rotator."
            n15 = stacked-sequence "Level-4, flat sequence structure, inside the case structure, starts a sequence of unit initialization." {
              tunnel: w55 -> [w56 _ _ _]
              tunnel: w54 -> [_ _ _ w111]
              frame #0 {
                n16 = flat-sequence {
                  tunnel: [w60] -> w58
                  tunnel: [w59] -> w57
                  tunnel: w56 -> [w59]
                  tunnel: w58 -> [w66]
                  tunnel: w57 -> [w64]
                  frame #0 {
                    n17 = property on="Keithley status" class="Bool (strict)"("Value"=FALSE ("Keithley status")) -> (error out=w62:errorcluster)  [unwired: 2 in, 1 out]
                    n18 = property on="Initial devices" class="Bool"(error in=w62, "Caption.Text"="Keithley...") -> (error out=w60:errorcluster)  [unwired: 1 in, 1 out]
                  }
                  frame #1 {
                    n19 = call "Initialize.vi"("error in (no error)"=w66, "VISA resource name"=w64) -> ("error out"=w65:errorcluster)  [unwired: 8 in, 1 out]
                    n20 = Unbundle By Name(w65) -> ("status"=w68:bool)
                    n21 = Not(x=w68) -> (.not. x?=→"Keithley status":bool)
                  }
                  frame #2 {
                    n22 = Wait (ms)(milliseconds to wait=u32 1000) -> ()  [unwired: 1 out]
                  }
                }
              }
              frame #1 {
                n23 = flat-sequence {
                  frame #0 {
                    # "YJ@Message, reminding that the monochromator is being initialized."
                    n24 = property on="Mono status" class="Bool (strict)"("Value"=FALSE ("Mono status")) -> (error out=w70:errorcluster)  [unwired: 2 in, 1 out]
                    n25 = property on="Initial devices" class="Bool"(error in=w70, "Caption.Text"="Monochromator...") -> ()  [unwired: 1 in, 2 out]
                  }
                  frame #1 {
                    # "YJ@ First Initialize the Monochomator, then move to the Start Wavelength Position."
                    n26 = Path To String(path="MC Config File (19523)") -> (string=w74:string)
                    n27 = call "LOT_System_Setup.vi"("CFG File Path"=w74) -> ()  [unwired: 2 in, 1 out]
                    "Mono status" <- TRUE
                  }
                  frame #2 {
                    n28 = local read "Start Wavelength (nm)"() -> (w77:sgl)
                    n29 = call "LOT_Select_Wavelength.vi"("Input Wavelength"=w77) -> ("Current Wavelength"=→"Current Wavelength":dbl)  [unwired: 1 out]
                  }
                }
              }
              frame #2 {
                n30 = flat-sequence {
                  frame #0 {
                    n31 = property on="Lockin status" class="Bool (strict)"("Value"=FALSE ("Mono status")) -> (error out=w78:errorcluster)  [unwired: 2 in, 1 out]
                    n32 = property on="Initial devices" class="Bool"(error in=w78, "Caption.Text"="Lock-in...") -> ()  [unwired: 1 in, 2 out]
                  }
                  frame #1 {
                    # "YJ@After Initialization, \n1) Time Constant is set to be 100 ms;\n2) Sensitivity is set to be 1 V;"
                    # "YJ@ \n1) FMOD, Set (Query) the Reference Source to External (0) or Internal (1).\n2) RSLP, set the External Reference Slope to Sine(0), TTL Rising (1), or TTL Falling (2)."
                    # "YJ@ from VISA address to GPIB:\n1) VISA, GPIB0::8::INSTR;\n2) GPIB, 0:8."
                    n33 = Unbundle By Name("lockin") -> ("Lock-in VISA address"=w92:refnum<visa-resource-name>)
                    n34 = call "Initialize.vi"("error in (no error)"=errorcluster {"status"=FALSE, "code"=0, "source"=""}, "VISA resource name"=w92) -> ("error out"=w85:errorcluster, "VISA resource name out"=w82:refnum<visa-resource-name>)  [unwired: 8 in]
                    n35 = property class="Instr"(reference=w82) -> ("Intf Num"=w91:u16, "Primary Addr"=w87:u16)  [unwired: 1 in, 2 out]
                    n36 = VISA Write(VISA resource name=w82, write buffer="FMOD0;RSLP2", error in (no error)=w85) -> (error out=w81:errorcluster)  [unwired: 2 out]
                    n37 = Unbundle By Name(w81) -> ("status"=w94:bool)
                    n38 = Not(x=w94) -> (.not. x?=→"Lockin status":bool)
                    n39 = Number To Decimal String(number=w91) -> (decimal integer string=w89:string)  [unwired: 1 in]
                    n40 = Number To Decimal String(number=w87) -> (decimal integer string=w86:string)  [unwired: 1 in]
                    n41 = Concatenate Strings(w89, ":" ("string"), w86) -> (→"GPIB address":string)
                  }
                  frame #2 {
                    n42 = Wait (ms)(milliseconds to wait=u32 1000) -> ()  [unwired: 1 out]
                  }
                }
              }
              frame #3 {
                # "YJ@Ignor the rever and forward limit switch, so the rotator can move in both directions."
                # "YJ@ \n1, No Error, True, Execute;\n0, Error, False;"
                # "YJ@ Avoid endless Initialization.\n1) Include the Initialization Process in the case structure."
                # "YJ@This APT homing subVI only execute when the motor is not at home."
                # "YJ@this output is always zero."
                # "YJ@Motor homed (1 - homed, 0 - not homed)."
                # "YJ@LED is light if there is No Error AND Motor Moved Home."
                # "YJ@ After no:\n0 for Error;\n1 for No Error;"
                # "YJ@ Frame-3, Initialize Rotator."
                n43 = property on="Rotator status" class="Bool (strict)"(error in=errorcluster {"status"=FALSE, "code"=0, "source"=""} ("error in (no error)"), "Value"=FALSE ("x .and. y?")) -> (error out=w115:errorcluster)  [unwired: 1 in, 1 out]
                n44 = property on="Initial devices" class="Bool"(error in=w115, "Caption.Text"="Rotator...") -> (error out=w97:errorcluster)  [unwired: 1 in, 1 out]
                n45 = property class="BenchtopStepperControl"(reference=w111, error in=w97, "SerialNumber"="40846753") -> (reference out=w109:refnum<k24>)  [unwired: 1 out]
                n46 = invoke class="BenchtopStepperControl" method="CreateDevice"(reference=w109) -> (reference out=w108:refnum<k24>)  [unwired: 2 in, 2 out]
                n47 = property class="BenchtopStepperControl"(reference=w108) -> (error out=w106:errorcluster, "BenchtopStepperMotor"=w107:refnum<k24>)  [unwired: 1 in, 1 out]
                "BenchtopStepperMotor" <- w107
                n48 = call "Kinesis Home.vi"("error in (no error)"=w106, ".NET Refnum in"=w107) -> ("error out"=w104:errorcluster, ".NET Refnum out"=w105:refnum<k24>)  [unwired: 8 in]
                n49 = call "Kinesis Move.vi"("error in (no error)"=w104, "Move Position"=0.0, ".NET Refnum in"=w105) -> ("error out"=w101:errorcluster, "Position"=→"Current degree":dbl)  [unwired: 7 in]
                n50 = Unbundle By Name(w101) -> ("status"=w100:bool)
                n51 = Not(x=w100) -> (.not. x?=→"Rotator status":bool)
                n52 = property on="Position of filter 1" class="DigNum (strict)"() -> ("Value"=w112:dbl)  [unwired: 2 in, 2 out]
                n53 = Divide(x=w112, y=360.0) -> ()  [unwired: 1 out]
                n54 = property on="Initial devices" class="Bool"(error in=w101, "Caption.Text"="Initialization completed") -> ()  [unwired: 1 in, 2 out]
              }
            }
          }
        }
        n55 = case "Level-3, case structure, controlled by an OK buttong, determine whether to Anticlosewisely rotate the rotator." shown="True" "Anticlockwise" {
          frame False {
          }
          frame True {
            n56 = property on="Current degree" class="DigNum (strict)"() -> ("Value"=w51:dbl)  [unwired: 2 in, 2 out]
            n57 = local read "BenchtopStepperMotor"() -> (w47:refnum<k24>)
            n58 = Fract/Exp String To Number(string="Step") -> (number=w52:dbl)  [unwired: 3 in, 1 out]
            n59 = Add(x=w51, y=w52) -> (x+y=w48:dbl)
            n60 = call "Kinesis Move.vi"("error in (no error)"=errorcluster {"status"=FALSE, "code"=0, "source"=""}, "Move Position"=w48, ".NET Refnum in"=w47) -> ("error out"=w44:errorcluster, "Position"=w45:dbl)  [unwired: 7 in]
            n61 = Unbundle By Name(w44) -> ("status"=w50:bool)
            n62 = Not(x=w50) -> (.not. x?=w49:bool)
            n63 = property on="Current degree" class="DigNum (strict)"(error in=w44, "Value"=w45) -> ()  [unwired: 1 in, 2 out]
            n64 = property on="Rotator status" class="Bool (strict)"("Value"=w49) -> ()  [unwired: 2 in, 2 out]
          }
        }
        n65 = property on="Position of filter 1" class="DigNum (strict)"() -> ("Value"=w24:dbl)  [unwired: 2 in, 2 out]
        n66 = property on="Current degree" class="DigNum (strict)"() -> ("Value"=w25:dbl)  [unwired: 2 in, 2 out]
        n67 = Subtract(x=w24, y=w25) -> (x-y=w23:dbl)
        n68 = Divide(x=w23, y=60.0) -> (x/y=w22:dbl)
        n69 = case "Level-3, case structure, controlled by an OK buttong, determine whether to Closewisely rotate the rotator." shown="True" "clockwise" {
          frame False {
          }
          frame True {
            n70 = property on="Current degree" class="DigNum (strict)"() -> ("Value"=w42:dbl)  [unwired: 2 in, 2 out]
            n71 = property on="Step" class="CmbBox"() -> ("Value"=w43:string)  [unwired: 2 in, 2 out]
            n72 = Fract/Exp String To Number(string=w43) -> (number=w41:dbl)  [unwired: 3 in, 1 out]
            n73 = Subtract(x=w42, y=w41) -> (x-y=w36:dbl)
            n74 = local read "BenchtopStepperMotor"() -> (w37:refnum<k24>)
            n75 = call "Kinesis Move.vi"("error in (no error)"=errorcluster {"status"=FALSE, "code"=0, "source"=""}, "Move Position"=w36, ".NET Refnum in"=w37) -> ("error out"=w34:errorcluster, "Position"=w33:dbl)  [unwired: 7 in]
            n76 = property on="Current degree" class="DigNum (strict)"(error in=w34, "Value"=w33) -> (error out=w40:errorcluster)  [unwired: 1 in, 1 out]
            n77 = Unbundle By Name(w40) -> ("status"=w39:bool)
            n78 = Not(x=w39) -> (.not. x?=w38:bool)
            n79 = property on="Rotator status" class="Bool (strict)"("Value"=w38) -> ()  [unwired: 2 in, 2 out]
          }
        }
        n80 = Round Toward +Infinity(x=w22) -> (ceil(x): smallest int >= x=w21:dbl)
        n81 = property on="Current Filter" class="DigNum (strict)"("Value"=w21) -> ()  [unwired: 2 in, 2 out]
        n82 = case "Level-3, case structure, to set a value to be the position of filter-1." shown="True" "Set as filter 1" {
          frame False {
          }
          frame True {
            n83 = property on="Current degree" class="DigNum (strict)"() -> ("Value"=→"Position of filter 1":dbl)  [unwired: 2 in, 2 out]
          }
        }
        n84 = case "Level-3, case structure, controlled by OK buttong, determine whether to Start Experiments." shown="True" "Start EXP" {
          tunnel: w31 -> [_ w118]
          frame False {
          }
          frame True {
            # "YJ@Start Exp:\nFrame-0, Initialize empty arrays to be used for data store. \nFrame-1, set up wavelength range & load calibaration files.\nFrame-2,\nFrame-3,"
            n85 = stacked-sequence "Level-4, flat sequence structure, inside the Start Exp case structure, and run the experiment following a sequence of actions," {
              tunnel: w118 -> [w123 _ _ w379]
              frame #0 {
                w121 = 0
                # "YJ@Set up empty arrays"
                # "YJ@Apply bias if desired"
                n86 = local read "Use Keithley for Bias?"() -> (w119:bool)
                n87 = Initialize Array "Initialize Array"(w121, w121) -> (w122:i32[])
                "EQE data" <- w122
                n88 = property on="Delay (s)" class="DigNum (strict)"() -> ("Value"=w120:sgl)  [unwired: 2 in, 2 out]
                n89 = case shown="True" w119 {
                  tunnel: w120 -> [_ w133]
                  tunnel: "Bias (V)" -> [_ w129]
                  tunnel: [errorcluster {"status"=FALSE, "code"=0, "source"=""} ("error out") w131] -> w125
                  tunnel: w123 -> [_ w127]
                  frame False {
                  }
                  frame True {
                    w128 = 0.1
                    w134 = 1
                    n90 = Multiply(x=1000, y=w133) -> (x*y=w141:sgl)
                    n91 = Wait (ms)(milliseconds to wait=w141) -> ()  [unwired: 1 out]
                    n92 = call "keithley_init.vi"("Displayed Measurement (0: Voltage)"=w134, "Measure Function (0: Volts)"=w134, "Enable Voltage Auto Range (T:Enable)"=FALSE ("Enable Output (T: Enable)"), "Output Level (0)"=w129, "Compliance  Level (0.1)"=w128, "Source Mode  (0: Voltage)"=0, "VISA resource name"=w127) -> ("error out"=w138:errorcluster, "VISA resource name out"=w137:refnum<visa-resource-name>)  [unwired: 3 in]
                    n93 = call "Enable Output.vi"("error in (no error)"=w138, "Enable Output (T: Enable)"=TRUE, "VISA resource name"=w137) -> ("error out"=w132:errorcluster, "VISA resource name out"=w130:refnum<visa-resource-name>)  [unwired: 7 in]
                    n94 = call "Configure Output.vi"("error in (no error)"=w132, "Compliance  Level (0.1)"=w128, "Output Level (0)"=w129, "VISA resource name"=w130) -> ("error out"=w131:errorcluster)  [unwired: 6 in, 1 out]
                  }
                }
                n95 = local write "Theta Device"(w122) -> ()
                n96 = local write "Device Current (A)"(w122) -> ()
                n97 = local write "Reference Current (A)"(w122) -> ()
                n98 = call <vilib>:"General Error Handler.vi"("error in (no error)"=w125) -> ()  [unwired: 10 in, 5 out]
              }
              frame #1 {
                # "YJ@ Frame-1, \n1) set up the wavelength range."
                # "Linear Interpolation of \ncalibration or\nphotodetector response"
                # "YJ@ Frame-1, \n2) Load in Calibration file or reference EQE."
                n99 = Build Array "Build Array"("Start Wavelength (nm)") -> (w152:sgl[])
                n100 = while {
                  shift-right: [w154] -> _
                  shift-left: w152 -> [w156]
                  tunnel: "Step size (nm)" -> [w163]
                  tunnel: "End Wavelength (nm)" -> [w164]
                  tunnel: "Start Wavelength (nm)" -> [w157]
                  tunnel: [w154] -> w143
                  i -> [w159]
                  stop <- w161 stop-if-true
                  # "Set up wavelenth array"
                  n101 = Multiply(x=w159, y=w163) -> (x*y=w162:sgl)
                  n102 = Add(x=w162, y=w157) -> (x+y=w155:sgl)
                  n103 = Greater Or Equal?(x=w155, y=w164) -> (x >= y?=w161:bool)
                  n104 = Equal?(x=w159, y=0) -> (x = y?=w158:bool)
                  n105 = case shown="False" w158 {
                    tunnel: w156 -> [w167 w168]
                    tunnel: w155 -> [w166 _]
                    tunnel: [w165 w168] -> w154
                    frame False {
                      n106 = Build Array (concatenate)(w167, w166) -> (w165:sgl[])
                    }
                    frame True {
                    }
                  }
                }
                "Wavelength range" <- w143
                n107 = case shown="\"Take Measurement\"" "FileIO" {
                  tunnel: [w170 w180] -> w149
                  tunnel: [w171 w181] -> w148
                  tunnel: w143 -> [_ w178]
                  frame "Take Calibration", Default {
                    # "Load Photodetector response for calibration scan"
                    n108 = call-poly <vilib>:"Read From Spreadsheet File.vi"("file path (dialog if empty)"="Load Calibration Reference file") -> ("all rows"=w175:dbl[][])  [unwired: 6 in, 4 out]
                    n109 = Index Array(array=w175, index (col)=0) -> (element=w171:dbl[])  [unwired: 1 in]
                    n110 = Index Array(array=w175, index (col)=1) -> (element=w170:dbl[])  [unwired: 1 in]
                    n111 = Bundle("all rows"=w171, "all rows"=w170) -> (→"YJ@ KSC photodetector_Si_KSC.txt":cluster{"all rows":dbl[], "all rows":dbl[]})  [unwired: 1 in]
                  }
                  frame "Take Measurement" {
                    # "YJ@ Load Calibration File"
                    n112 = call-poly <vilib>:"Read From Spreadsheet File.vi"("file path (dialog if empty)"="AM1p5_1sun_photoflux") -> ("all rows"=w190:dbl[][])  [unwired: 6 in, 4 out]
                    n113 = call-poly <vilib>:"Read From Spreadsheet File.vi"("file path (dialog if empty)"="70356_70316NS_473.txt") -> ("all rows"=w191:dbl[][])  [unwired: 6 in, 4 out]
                    n114 = Index Array(array=w190, index (col)=0 ("disabled index (col)")) -> (element=w185:dbl[])  [unwired: 1 in]
                    n115 = Index Array(array=w190, index (col)=1 ("disabled index (col)")) -> (element=w184:dbl[])  [unwired: 1 in]
                    n116 = Index Array(array=w191, index (col)=0) -> (element=w181:dbl[])  [unwired: 1 in]
                    n117 = Index Array(array=w191, index (col)=1) -> (element=w180:dbl[])  [unwired: 1 in]
                    n118 = Bundle("all rows"=w181, "all rows"=w180) -> (→"70356_70316NS_473.txt":cluster{"all rows":dbl[], "all rows":dbl[]})  [unwired: 1 in]
                    n119 = Bundle("all rows"=w185, "all rows"=w184) -> (→"YJ@ AM1p5_1sun_photonflux":cluster{"all rows":dbl[], "all rows":dbl[]})  [unwired: 1 in]
                    n120 = call <vilib>:"Interpolate 1D.vi"("method"=1, "X is monotonic"=TRUE, "xi"=w178, "X"=w185, "Y"=w184) -> ("yi"=w177:dbl[])  [unwired: 4 in, 2 out]
                    "Photonflux" <- w177
                    n121 = Bundle(w178, "yi"=w177) -> (→"YJ@ AM1p5_1sun_photonflux_after interpolation":cluster{sgl[], "yi":dbl[]})  [unwired: 1 in]
                  }
                }
                n122 = call <vilib>:"Interpolate 1D.vi"("method"=1, "X is monotonic"=TRUE, "xi"=w143, "X"=w148, "Y"=w149) -> ("yi"=w153:dbl[])  [unwired: 4 in, 2 out]
                n123 = Bundle(w143, "yi"=w153) -> (→"70356_70316NS_473 File":cluster{sgl[], "yi":dbl[]})  [unwired: 1 in]
              }
              frame #2 {
                # "YJ@It behaves as a waiting time."
                # "YJ@Step-5, Start the measurement.\nWavelength point is fed one-by-one into the while loop."
                # "YJ@Step-4, Lock-in:\nSet the sensitivity according to the first signal at the presetted start wavelength and the time constant."
                # "YJ@Step-3, Lock-in:\nSet the time constant according to the Integration (ms)."
                # "YJ@ Set (Query) the Time Constant to 10 us (0) through 30 ks (19)."
                # "YJ@Lock-in time constant:\n1) the unit is ms;\n2) the actual minimum is 10 us, i.e. 0.01 ms;\n3) the actual maximum should be 30 s, i.e., 30 000 ms;"
                # "YJ@Step-2, Rotator:\nMove to the Filter-1 position."
                # "YJ@Step-1, Monochromator: Move to the Start Wavelength position."
                # "YJ@ 400, 410, 420."
                n124 = local read "Start Wavelength (nm)"() -> (w202:sgl)
                n125 = property on="Start EXP" class="Bool"("BoolText.Text"="Scanning" ("Caption.Text")) -> (error out=w200:errorcluster)  [unwired: 2 in, 1 out]
                n126 = call "LOT_Select_Wavelength.vi"("Input Wavelength"=w202) -> ("Current Wavelength"=w201:dbl)  [unwired: 1 out]
                n127 = property on="Current Wavelength" class="DigNum (strict)"(error in=w200, "Value"=w201) -> (error out=w210:errorcluster)  [unwired: 1 in, 1 out]
                n128 = local read "BenchtopStepperMotor"() -> (w199:refnum<k24>)
                n129 = property on="Position of filter 1" class="DigNum (strict)"(error in=w210) -> (error out=w198:errorcluster, "Value"=w197:dbl)  [unwired: 1 in, 1 out]
                n130 = call "Kinesis Move.vi"("error in (no error)"=w198, "Move Position"=w197, ".NET Refnum in"=w199) -> ("error out"=w195:errorcluster, "Position"=w196:dbl)  [unwired: 7 in]
                n131 = property on="Current degree" class="DigNum (strict)"(error in=w195, "Value"=w196) -> (error out=w209:errorcluster)  [unwired: 1 in, 1 out]
                n132 = property on="lockin" class="Clust (strict)"(error in=w209) -> (error out=w217:errorcluster, "Value"=w226:T2)  [unwired: 1 in, 1 out]
                n133 = Unbundle By Name(w226) -> ("Lock-in VISA address"=w216:refnum<visa-resource-name>, "Integration (ms)"=w206:u32)
                n134 = Divide(x=w206, y=u32 10) -> (x/y=w204:dbl)
                n135 = Divide(x=w204, y=dbl[] [0.01, 0.03, 0.1, 0.3, 1.0, 3.0, 10.0, 30.0, 100.0, 300.0, 1000.0, 3000.0, 10000.0, 30000.0, 100000.0, 300000.0, 1000000.0, 3000000.0, 10000000.0, 30000000.0]) -> (x/y=w224:dbl[])
                n136 = Round Toward +Infinity(x=w224) -> (ceil(x): smallest int >= x=w223:dbl[])
                n137 = Search 1D Array(1D array=w223, element=1.0) -> (index of element=w219:i32)  [unwired: 1 in]
                n138 = Number To Decimal String(number=w219) -> (decimal integer string=w218:string)  [unwired: 1 in]
                n139 = Concatenate Strings "Concatenate Strings"("OFLT" ("string"), w218) -> (w221:string)
                n140 = VISA Write(VISA resource name=w216, write buffer=w221, error in (no error)=w217) -> (VISA resource name out=w215:refnum<visa-resource-name>, error out=w212:errorcluster)  [unwired: 1 out]
                n141 = property on="Auto Scale" class="Str"(error in=w212, "Value"="Scaling..." ("Auto sclae")) -> (error out=w211:errorcluster)  [unwired: 1 in, 1 out]
                n142 = Divide(x=w206, y=u32 3) -> (x/y=w207:dbl)
                n143 = call "Lockin_autoscale.vi"("error in (no error)"=w211, "Integration time (ms)"=w207, "VISA resource name"=w215) -> ("error out"=w208:errorcluster, "String"=w214:string)  [unwired: 1 in, 1 out]
                n144 = property on="Auto Scale" class="Str"("Value"=w214) -> ()  [unwired: 2 in, 2 out]
                n145 = local read "Wavelength range"() -> (w229:sgl[])
                n146 = Array Size(array=w229) -> (size(s)=w228:i32)
                n147 = while "Level-5, while loop, Start wavelength by wavelength measurements." {
                  tunnel: w229 -> [w253] mode=indexing
                  tunnel: w228 -> [w252]
                  tunnel: w208 -> [w239]
                  i -> [w251]
                  stop <- w247 stop-if-true
                  # "YJ@stop the measurement when all wavelength points are maesured."
                  # "Scan through wavelengths, make measurement and update graph"
                  n148 = Increment(x=w251) -> (x+1=w250:i32)
                  n149 = Greater Or Equal?(x=w250, y=w252) -> (x >= y?=w248:bool)
                  n150 = flat-sequence {
                    tunnel: w251 -> [w265]
                    tunnel: [w265] -> w238
                    tunnel: w253 -> [w263]
                    tunnel: [w263] -> w237
                    tunnel: w248 -> [w264]
                    tunnel: [w264] -> w236
                    tunnel: w239 -> [_]
                    tunnel: w238 -> [w279]
                    tunnel: [w279] -> w235
                    tunnel: w237 -> [w271]
                    tunnel: [w271] -> w233
                    tunnel: w236 -> [w278]
                    tunnel: [w278] -> w231
                    tunnel: w235 -> [w282]
                    tunnel: [w282] -> w234
                    tunnel: w233 -> [w281]
                    tunnel: [w281] -> w232
                    tunnel: w231 -> [w280]
                    tunnel: [w280] -> w230
                    tunnel: [w325] -> w243
                    tunnel: [w323] -> w242
                    tunnel: w234 -> [w318]
                    tunnel: [w318] -> w241
                    tunnel: w232 -> [w319]
                    tunnel: w230 -> [w296]
                    tunnel: [w296] -> w240
                    tunnel: [w352] -> w259
                    tunnel: w243 -> [w352]
                    tunnel: [w351] -> w257
                    tunnel: w242 -> [w351]
                    tunnel: [w359] -> w255
                    tunnel: w241 -> [w366]
                    tunnel: w240 -> [w354]
                    tunnel: [w353] -> w247
                    frame #0 {
                      # "YJ@step-1, move the Mono-chronomator."
                      # "Pause Lock in measurement if requested"
                      # "Go to wavelength"
                      n151 = while {
                        stop <- w267 stop-if-true
                        n152 = Not(x="Pause Request") -> (.not. x?=w267:bool)
                        n153 = Wait (ms)(milliseconds to wait=u32 20) -> ()  [unwired: 1 out]
                        "Paused" <- "Pause Request"
                      }
                      n154 = call "LOT_Select_Wavelength.vi"("Input Wavelength"=w263) -> ("Current Wavelength"=w262:dbl)  [unwired: 1 out]
                      n155 = local write "Current Wavelength"(w262) -> ()
                    }
                    frame #1 {
                      # "YJ@wavelength"
                      # "YJ@ step-2, move the Filter wheel accordingly."
                      n156 = property on="Position of filter 1" class="DigNum (strict)"() -> ("Value"=w270:dbl)  [unwired: 2 in, 2 out]
                      n157 = local read "BenchtopStepperMotor"() -> (w269:refnum<k24>)
                      n158 = call "Kinesis clockwise move.vi"("degree of filter 1"=w270, "wavelength"=w271, ".NET Refnum in"=w269) -> ("GetPosition_Position"=w276:sgl, "error out"=w277:errorcluster)  [unwired: 7 in]
                      n159 = Subtract(x=w270, y=w276) -> (x-y=w274:dbl)
                      n160 = property on="Current degree" class="DigNum (strict)"(error in=w277, "Value"=w276) -> ()  [unwired: 1 in, 2 out]
                      n161 = Divide(x=w274, y=60.0) -> (x/y=w272:dbl)
                      n162 = Round Toward +Infinity(x=w272) -> (ceil(x): smallest int >= x=→"Current Filter":dbl)
                    }
                    frame #2 {
                      # "YJ@possible waiting time before data acquisition."
                    }
                    frame #3 {
                      # "YJ@Auto scaling, select a propriate sensitivity."
                      # "YJ@wavelength."
                      # "YJ@ Reference Value"
                      # "1.5 (s)"
                      # "YJ@ Device Value."
                      # "YJ@ This value was 5 before, meaning autogain is activated every 5 points."
                      # "Add to Array of current\nmeasurements"
                      # "YJ@Measure current"
                      n163 = Quotient & Remainder(x=w318, y="Auto Gain Point Separation") -> (x-y*floor(x/y)=w305:i32)  [unwired: 1 out]
                      n164 = Greater?(x=w319, y="Autoscale Starts") -> (0:w303:bool)
                      n165 = Equal To 0?(x=w305) -> (x = 0?=w304:bool)
                      n166 = And(x=w304, y=w303) -> (x .and. y?=w290:bool)
                      n167 = property on="lockin" class="Clust (strict)"() -> (error out=w289:errorcluster, "Value"=w288:T2)  [unwired: 2 in, 1 out]
                      n168 = And(x=w290, y="Autogain") -> (x .and. y?=w286:bool)
                      n169 = case shown="False" w286 {
                        tunnel: [w326 w330] -> w291
                        tunnel: w289 -> [w326 w334]
                        tunnel: w288 -> [_ w336]
                        frame False {
                        }
                        frame True {
                          n170 = Unbundle By Name(w336) -> ("Lock-in VISA address"=w331:refnum<visa-resource-name>, "Integration (ms)"=w329:u32)
                          n171 = property on="Auto Scale" class="Str"(error in=w334, "Value"="Scaling..." ("Auto sclae")) -> (error out=w333:errorcluster)  [unwired: 1 in, 1 out]
                          n172 = Divide(x=w329, y=u32 3) -> (x/y=w327:dbl)
                          n173 = call "Lockin_autoscale.vi"("error in (no error)"=w333, "Integration time (ms)"=w327, "VISA resource name"=w331) -> ("error out"=w330:errorcluster, "String"=→"Auto Scale":string)  [unwired: 1 in, 1 out]
                        }
                      }
                      n174 = property on="lockin" class="Clust (strict)"() -> ("Value"=w295:T2)  [unwired: 2 in, 2 out]
                      n175 = Unbundle By Name(w295) -> ("Integration (ms)"=w293:u32, "data storage rate (Hz)"=w294:T7)
                      n176 = property on="GPIB address" class="Str"() -> ("Value"=w292:string)  [unwired: 2 in, 2 out]
                      n177 = Multiply(x=1000.0, y="Delay-2 (s)") -> (x*y=w301:dbl)
                      n178 = call "TakeDatafrom2_SR830lockins.vi"("Reference Dector Lockin Address"="Ref. Detector\nLockin Address", "Device Lockin Address"=w292, "Delay (ms)"=w301, "Integration (ms)"=w293, "data storage rate (Hz)"=w294, "error in"=w291, "Use Reference Detector"="Use Reference Detector", "Mean (T) or Median (F)"="Average Method", "Measure Mode\n(T =Signal)"=TRUE ("Average Method")) -> ("Device value (complex)"=w310:cdb, "Reference value (complex)"=w312:cdb, "error out"=w308:T8)  [unwired: 3 in, 1 out]
                      n179 = Complex To Polar(r * e^(i*theta)=w310) -> (r=w309:dbl, theta=w320:dbl)
                      n180 = Complex To Polar(r * e^(i*theta)=w312) -> (r=w311:dbl)  [unwired: 1 out]
                      n181 = local read "Gain (ohms, ref)"() -> (w313:dbl)
                      n182 = local read "Gain (ohms, device)"() -> (w317:dbl)
                      n183 = local read "Theta Device"() -> (w321:dbl[])
                      n184 = Build Array (concatenate) "Build Array"(w321, w320) -> (w297:dbl[])
                      n185 = Divide(x=w309, y=w317) -> (x/y=w299:dbl)
                      n186 = Divide(x=w311, y=w313) -> (x/y=w300:dbl)
                      n187 = local write "Theta Device"(w297) -> ()
                      n188 = case shown="True" FALSE {
                        tunnel: w292 -> [_ w342]
                        tunnel: w308 -> [w337 w341]
                        tunnel: [w337 w340] -> w307
                        tunnel: "Delay-2 (s)" -> [_ w339]
                        tunnel: w290 -> [_ w338]
                        frame False {
                        }
                        frame True {
                          n189 = case shown="False" w338 {
                            tunnel: w342 -> [_ w349]
                            tunnel: w341 -> [w343 w348]
                            tunnel: [w343 w344] -> w340
                            tunnel: w339 -> [_ w346]
                            frame False {
                            }
                            frame True {
                              n190 = GPIB Write(0:w349, 1:"AGAN;", 3:w348) -> (6:w345:errorcluster)  [unwired: 2 in, 1 out]
                              n191 = call "Time Delay2"("error in (no error)"=w345, "Delay Time (s)"=w346) -> ("error out"=w344:errorcluster)  [unwired: 9 in]
                            }
                          }
                        }
                      }
                      n192 = local read "Reference Current (A)"() -> (w322:dbl[])
                      n193 = local read "Device Current (A)"() -> (w324:dbl[])
                      n194 = Build Array (concatenate)(w324, w299) -> (w325:dbl[])
                      n195 = Build Array (concatenate)(w322, w300) -> (w323:dbl[])
                      n196 = local write "Reference Current (A)"(w323) -> ()
                      n197 = local write "Device Current (A)"(w325) -> ()
                      n198 = call <vilib>:"Simple Error Handler.vi"("error in (no error)"=w307) -> ()  [unwired: 4 in, 5 out]
                    }
                    frame #4 {
                      # "Calibration scan:\nCalibration = device photodiode/ ref photodiode\n              / device photodiode spec"
                      # "EQE= Device Current/Ref Photodiode / Calibration"
                      # "Calculate EQE"
                      n199 = local read "70356_70316NS_473 File"() -> (w350:cluster{sgl[], "yi":dbl[]})
                      n200 = local read "Reference Current (A)"() -> (w356:dbl[])
                      n201 = local read "Device Current (A)"() -> (w357:dbl[])
                      n202 = Or(x=w354, y="stop 3") -> (x .or. y?=w353:bool)
                      n203 = Index Array "Index Array"(array=w357, index=w366) -> (element=w365:dbl)
                      n204 = Index Array(array=w356, index=w366) -> (element=w364:dbl)
                      n205 = Unbundle(w350) -> ("yi"=w360:dbl[])  [unwired: 1 out]
                      n206 = Index Array(array=w360, index=w366) -> (element=w362:dbl)
                      n207 = Divide(x=w365, y=w364) -> (x/y=w363:dbl)
                      n208 = Divide(x=w363, y=w362) -> (x/y=w361:dbl)
                      n209 = local read "EQE data"() -> (w358:dbl[])
                      n210 = Build Array (concatenate)(w358, w361) -> (w359:dbl[])
                      n211 = local write "EQE data"(w359) -> ()
                    }
                  }
                  n212 = Absolute Value(x=w259) -> (abs(x)=w258:dbl[])
                  n213 = Absolute Value(x=w255) -> (abs(x)=w244:dbl[])
                  n214 = Absolute Value(x=w257) -> (abs(x)=w256:dbl[])
                  n215 = local read "FileIO"() -> (w246:enum32{"Take Calibration", "Take Measurement"})
                  n216 = local read "Wavelength range"() -> (w254:sgl[])
                  n217 = case shown="\"Take Measurement\"" w246 {
                    tunnel: [0.0 w369] -> w245
                    tunnel: w244 -> [_ w368]
                    frame "Take Calibration", Default {
                    }
                    frame "Take Measurement" {
                      n218 = local read "Step size (nm)"() -> (w371:sgl)
                      n219 = local read "Photonflux"() -> (w372:dbl[])
                      n220 = for {
                        tunnel: w372 -> [w376] mode=indexing
                        tunnel: w368 -> [w377] mode=indexing
                        tunnel: w371 -> [w374]
                        tunnel: [w373] -> w370 mode=indexing
                        n221 = Multiply(x=w376, y=w377) -> (x*y=w375:dbl)
                        n222 = Multiply(x=w374, y=w375) -> (x*y=w373:dbl)
                      }
                      n223 = Add Array Elements(numeric array=w370) -> (sum=w369:dbl)
                    }
                  }
                  "Integrated Photocurrent (mA/cm2):" <- w245
                  n224 = Bundle("Wavelength range"=w254, w258) -> (→"Device Current":cluster{"Wavelength range":sgl[], dbl[]})  [unwired: 1 in]
                  n225 = Bundle("Wavelength range"=w254, w244) -> (→"EQE" →"EQE (log scale)":cluster{"Wavelength range":sgl[], dbl[]})  [unwired: 1 in]
                  n226 = Bundle("Wavelength range"=w254, w256) -> (→"Lamp Reference Photodetector Current":cluster{"Wavelength range":sgl[], dbl[]})  [unwired: 1 in]
                }
              }
              frame #3 {
                n227 = flat-sequence {
                  tunnel: w379 -> [w381]
                  tunnel: [w381] -> w378
                  tunnel: w378 -> [w382]
                  frame #0 {
                    n228 = property on="Start EXP" class="Bool"("BoolText.Text"="Start EXP" ("Caption.Text")) -> ()  [unwired: 2 in, 2 out]
                  }
                  frame #1 {
                    n229 = case shown="True" "Use Keithley for Bias?" {
                      tunnel: w382 -> [_ w384]
                      frame False {
                      }
                      frame True {
                        n230 = call "Configure Output.vi"("VISA resource name"=w384) -> ("error out"=w385:errorcluster, "VISA resource name out"=w386:refnum<visa-resource-name>)  [unwired: 9 in]
                        n231 = call "Enable Output.vi"("error in (no error)"=w385, "Enable Output (T: Enable)"=FALSE, "VISA resource name"=w386) -> ("error out"=w388:errorcluster, "VISA resource name out"=w389:refnum<visa-resource-name>)  [unwired: 7 in]
                        n232 = call "Close.vi"("error in (no error)"=w388, "VISA resource name"=w389) -> ("error out"=w390:errorcluster)  [unwired: 9 in]
                        n233 = call <vilib>:"General Error Handler.vi"("error in (no error)"=w390) -> ()  [unwired: 10 in, 5 out]
                      }
                    }
                  }
                  frame #2 {
                    w408 = TRUE
                    # "Save File and return monocromator to zero for white light"
                    n234 = local read "Integrated Photocurrent (mA/cm2):"() -> (w409:dbl)
                    n235 = local read "Bias (V)"() -> (w397:dbl)
                    n236 = Number To Fractional String(number=w397) -> (F-format string=w396:string)  [unwired: 3 in]
                    n237 = Number To Fractional String(number=w409) -> (F-format string=w410:string)  [unwired: 3 in]
                    n238 = local read "FileIO"() -> (w411:enum32{"Take Calibration", "Take Measurement"})
                    n239 = case shown="\"Take Measurement\"" w411 {
                      tunnel: [w415 w426] -> w413
                      tunnel: w410 -> [_ w424]
                      tunnel: w396 -> [_ w422]
                      frame "Take Calibration", Default {
                        n240 = Build Array "Build Array"("Wavelength (nm)", "Calibration", "Ref photodetector Current (A)", "Photodetector Current (A)", "Ref photodetector EQE") -> (w415:string[])
                      }
                      frame "Take Measurement" {
                        n241 = Build Array "Build Array"("Wavelength (nm)", "EQE (or reflectance)", "Device Current (A)", "Photodetector Current (A)", "Calibration", "Theta Device (for lockin measurement)", "Bias (V):", w422, "AM1.5 1sun (mA/cm2):", w424) -> (w426:string[])
                      }
                    }
                    n242 = local read "Lamp Reference Photodetector Current"() -> (w402:cluster{"Wavelength range":sgl[], dbl[]})
                    n243 = call-poly <vilib>:"Write To Spreadsheet File.vi"("1D data"=w413) -> ("new file path (Not A Path if cancelled)"=w412:path)  [unwired: 7 in]
                    n244 = local read "70356_70316NS_473 File"() -> (w401:cluster{sgl[], "yi":dbl[]})
                    n245 = local read "Theta Device"() -> (w392:dbl[])
                    n246 = local read "Device Current"() -> (w403:cluster{"Wavelength range":sgl[], dbl[]})
                    n247 = local read "EQE"() -> (w406:cluster{"Wavelength range":sgl[], dbl[]})
                    n248 = Divide(x=180, y=3.141592653589793) -> (x/y=w393:dbl)
                    n249 = Unbundle(w406) -> ("Wavelength range"=w405:sgl[], w404:dbl[])
                    n250 = Unbundle(w401) -> ("yi"=w398:dbl[])  [unwired: 1 out]
                    n251 = Unbundle(w403) -> (w400:dbl[])  [unwired: 1 out]
                    n252 = Unbundle(w402) -> (w399:dbl[])  [unwired: 1 out]
                    n253 = Multiply(x=w392, y=w393) -> (x*y=w391:dbl[])
                    n254 = Build Array "Build Array"(w405, w404, w400, w399, w398, w391) -> (w407:dbl[][])
                    n255 = call-poly <vilib>:"Write To Spreadsheet File.vi"("transpose? (no:F)"=w408, "format (%.3f)"="%g", "append to file? (new file:F)"=w408, "2D data"=w407, "file path (dialog if empty)"=w412) -> ()  [unwired: 3 in, 1 out]
                  }
                }
              }
            }
          }
        }
      }
      frame "Go To Wavelength" {
        n256 = flat-sequence {
          frame #0 {
            n257 = property on="Mono status" class="Bool (strict)"() -> ("Value"=w433:bool)  [unwired: 2 in, 2 out]
            n258 = property on="Current Wavelength" class="DigNum (strict)"() -> ("Value"=→"Current wavelength test (nm)":dbl)  [unwired: 2 in, 2 out]
            n259 = case shown="False" w433 {
              tunnel: [T6."Disabled and Grayed Out" ("Disabled") T6."Enabled" ("Disabled")] -> w432
              frame False {
              }
              frame True {
              }
            }
            n260 = property on="Goto wavelength" class="Bool"("DisabledEnum"=w432) -> ()  [unwired: 2 in, 2 out]
          }
          frame #1 {
            n261 = case shown="True" "Goto wavelength" {
              frame False {
              }
              frame True {
                n262 = flat-sequence {
                  frame #0 {
                    n263 = property on="Goto wavelength" class="Bool"("BoolText.Text"="Changing..." ("Boolean Text.Text")) -> ()  [unwired: 2 in, 2 out]
                  }
                  frame #1 {
                    n264 = call "LOT_Select_Wavelength.vi"("Input Wavelength"="Wavelength (nm)") -> ("Current Wavelength"=w439:dbl)  [unwired: 1 out]
                    n265 = local write "Current Wavelength"(w439) -> ()
                    n266 = property on="Goto wavelength" class="Bool"(error in=errorcluster {"status"=FALSE, "code"=0, "source"=""} ("error in (no error)"), "BoolText.Text"="Go to wavelength" ("Boolean Text.Text")) -> ()  [unwired: 1 in, 2 out]
                  }
                  frame #2 {
                  }
                }
              }
            }
          }
        }
      }
      frame "EQE(V)" {
        n267 = stacked-sequence {
          tunnel: "Lock-In IV curve calb tab" -> [w452 _ w584]
          tunnel: "Monochromator Controls" -> [w457 _ w582]
          tunnel: "Bias Parameters" -> [w456 w502 _]
          tunnel: "Lockin Parameters" -> [_ w503 w583]
          frame #0 {
            w465 = 1
            w471 = 0
            # "Set up Keithley 2400 for biasing"
            # "Go to wavelength"
            # "Set up arrays"
            n268 = Unbundle(w457) -> ("Wavelength (nm)"=w448:sgl)  [unwired: 1 out]
            n269 = Unbundle(w456) -> ("VISA resource name"=w462:refnum<visa-resource-name>, "Start Bias (V)"=w455:dbl, "End Bias (V)"=w461:dbl, "Number of points minus 1"=w460:i16, "Compliance (A)"=w449:dbl)
            n270 = call "Mono (YJ) - JPJ.vi"("Go to Wavelength"=w448) -> ("Current Wavelength"=w447:dbl)  [unwired: 3 in, 2 out]
            n271 = Format Value(format string=":CURR:RANG:AUTO 0; :CURR:RANG %s;", value (0)=w449) -> (output string=w453:string)  [unwired: 1 in]
            n272 = local write "Current Wavelength"(w447) -> ()
            n273 = case shown="\"Calibrate\", Default" w452 {
              tunnel: w455 -> [_ w481]
              tunnel: w461 -> [_ w480]
              tunnel: w460 -> [_ w479]
              tunnel: [w474 w475] -> w458
              tunnel: w455 -> [_ w477]
              tunnel: [w472 w476] -> w454
              tunnel: "Load Voltage Profile?" -> [_ w478]
              frame "Calibrate", Default {
                w472 = 0
                n274 = Initialize Array(w472, 1) -> (w474:i32[])
              }
              frame "Scan" {
                n275 = case shown="False" w478 {
                  tunnel: w481 -> [w487 _]
                  tunnel: w480 -> [w486 _]
                  tunnel: w479 -> [w483 _]
                  tunnel: w477 -> [w484 _]
                  tunnel: [w484 w495] -> w476
                  tunnel: [w485 w497] -> w475
                  frame False {
                    n276 = Equal To 0?(x=w483) -> (x = 0?=w482:bool)
                    n277 = case shown="False" w482 {
                      tunnel: w487 -> [w492 w494]
                      tunnel: w486 -> [w491 _]
                      tunnel: [w490 w493] -> w485
                      tunnel: w483 -> [w488 _]
                      frame False {
                        n278 = Increment(x=w488) -> (x+1=w489:i16)
                        n279 = call-poly <vilib>:"Ramp Pattern.vi"("start"=w492, "end"=w491, "samples"=w489) -> ("Ramp Pattern"=w490:dbl[])  [unwired: 7 in, 1 out]
                      }
                      frame True {
                        n280 = Build Array(w494) -> (w493:dbl[])
                      }
                    }
                  }
                  frame True {
                    w496 = 0
                    n281 = call-poly <vilib>:"Read From Spreadsheet File.vi"("file path (dialog if empty)"="Voltage Profile") -> ("all rows"=w498:dbl[][])  [unwired: 6 in, 4 out]
                    n282 = Index Array(array=w498, index (col)=w496) -> (element=w497:dbl[])  [unwired: 1 in]
                    n283 = Index Array(array=w497, index=w496) -> (element=w495:dbl)
                  }
                }
              }
            }
            "Applied Biases (V)" <- w458
            n284 = call "keithley_init.vi"("Displayed Measurement (0: Voltage)"=w465, "Measure Function (0: Volts)"=w465, "Enable Voltage Auto Range (T:Enable)"=TRUE ("Enable Output (T: Enable)"), "Output Level (0)"=w454, "Compliance  Level (0.1)"=w449, "Source Mode  (0: Voltage)"=0, "VISA resource name"=w462) -> ("error out"=w469:errorcluster, "VISA resource name out"=w468:refnum<visa-resource-name>)  [unwired: 3 in]
            n285 = call "Enable Output.vi"("error in (no error)"=w469, "Enable Output (T: Enable)"=TRUE, "VISA resource name"=w468) -> ("error out"=w463:errorcluster, "VISA resource name out"=w464:refnum<visa-resource-name>)  [unwired: 7 in]
            n286 = VISA Write(VISA resource name=w464, write buffer=w453, error in (no error)=w463) -> ()  [unwired: 3 out]
            n287 = Initialize Array(w471, w471) -> (→"Device Current (A)" →"DC current (A)" →"Reference Current (A)" →"Theta Device":i32[])
          }
          frame #1 {
            n288 = local read "Applied Biases (V)"() -> (w501:dbl[])
            n289 = Array Size(array=w501) -> (size(s)=w500:i32)
            n290 = while {
              tunnel: w501 -> [w512] mode=indexing
              tunnel: w503 -> [w511]
              tunnel: w502 -> [w510]
              tunnel: w500 -> [w507]
              i -> [w506]
              stop <- w508 stop-if-true
              n291 = Increment(x=w506) -> (x+1=w505:i32)
              n292 = stacked-sequence {
                tunnel: w512 -> [w517 _ _]
                tunnel: w510 -> [w513 w532 _]
                tunnel: w511 -> [_ w531 _]
                tunnel: [_ _ "stop 2"] -> w504
                frame #0 {
                  # "Apply Bias"
                  n293 = Unbundle(w513) -> ("VISA resource name"=w515:refnum<visa-resource-name>, "Compliance (A)"=w514:dbl)  [unwired: 3 out]
                  n294 = call "Configure Output.vi"("Compliance  Level (0.1)"=w514, "Output Level (0)"=w517, "VISA resource name"=w515) -> ("error out"=w516:errorcluster)  [unwired: 7 in, 1 out]
                  n295 = call <vilib>:"General Error Handler.vi"("error in (no error)"=w516) -> ()  [unwired: 10 in, 5 out]
                }
                frame #1 {
                  # "Measure Current"
                  # "For Device"
                  # "Lockin measurement"
                  n296 = local read "Gain (ohms, device)"() -> (w534:dbl)
                  n297 = Unbundle(w531) -> ("Device Lockin Address"=w557:string, "Wait (ms)"=w537:dbl, "Integration (ms)"=w556:u32, "data storage rate (Hz)"=w555:T7)  [unwired: 1 out]
                  n298 = Unbundle(w532) -> ("VISA resource name"=w533:refnum<visa-resource-name>)  [unwired: 4 out]
                  n299 = Divide(x=w537, y=1000) -> (x/y=w535:dbl)
                  n300 = call "Time Delay"("Delay Time (s)"=w535) -> ("error out"=w541:errorcluster)  [unwired: 10 in]
                  n301 = call-poly "Read.vi"("VISA resource name"=w533, "Sample Count (1)"=10, "error in (no error)"=w541) -> ("Current"=w539:sgl[], "error out"=w540:errorcluster)  [unwired: 6 in, 5 out]
                  n302 = case shown="True" "Use Reference Detector?" {
                    tunnel: [1 w568] -> w546
                    tunnel: w531 -> [_ w567]
                    tunnel: w541 -> [w559 w562]
                    tunnel: [w559 w561] -> w543
                    frame False {
                    }
                    frame True {
                      # "For Reference Detector"
                      n303 = Unbundle(w567) -> ("Ref. Lockin Address"=w566:string, "Integration (ms)"=w565:u32, "data storage rate (Hz)"=w564:T7)  [unwired: 2 out]
                      n304 = call "ReadandMedianSR830_ETH_copy2.vi"("data storage rate (Hz)"=0, "Lockin Address"=w566, "Integration (ms)"=w565, "Delay (ms)"=w564, "error in"=w562) -> ("signal (complex)"=w568:cdb, "error out"=w561:T8)  [unwired: 1 in, 1 out]
                    }
                  }
                  n305 = call-poly <vilib>:"Mean.vi"("X"=w539) -> ("mean"=w538:dbl)  [unwired: 1 out]
                  n306 = local read "DC current (A)"() -> (w549:dbl[])
                  n307 = call "ReadLockin_ETH_2median.vi"("Delay (ms)"=0, "Lockin Address"=w557, "Integration (ms)"=w556, "data storage rate (Hz)"=w555, "error in"=w541) -> ("R"=w528:dbl, "Theta (radians)"=w521:dbl, "error out"=w544:errorcluster)  [unwired: 1 in]
                  n308 = Polar To Re/Im(2:w521, 3:w528) -> (1:w530:dbl)  [unwired: 1 out]
                  n309 = Build Array (concatenate)(w549, w538) -> (w548:dbl[])
                  n310 = Sign(1:w530) -> (0:w529:dbl)
                  n311 = Multiply(x=w529, y=w528) -> (x*y=w527:dbl)
                  n312 = Divide(x=w527, y=w534) -> (x/y=w547:dbl)
                  n313 = local read "Gain (ohms, ref)"() -> (w519:dbl)
                  n314 = Merge Errors(w544, w543, w540) -> (w542:errorcluster)
                  n315 = local write "DC current (A)"(w548) -> ()
                  n316 = local read "Device Current (A)"() -> (w553:dbl[])
                  n317 = Divide(x=180, y=3.141592653589793) -> (x/y=w522:dbl)
                  n318 = Build Array (concatenate)(w553, w547) -> (w552:dbl[])
                  n319 = Divide(x=w546, y=w519) -> (x/y=w545:cdb)
                  n320 = Multiply(x=w521, y=w522) -> (x*y=w520:dbl)
                  n321 = local read "Theta Device"() -> (w526:dbl[])
                  n322 = call <vilib>:"General Error Handler.vi"("error in (no error)"=w542) -> ()  [unwired: 10 in, 5 out]
                  n323 = local write "Device Current (A)"(w552) -> ()
                  n324 = local read "Reference Current (A)"() -> (w551:dbl[])
                  n325 = Build Array (concatenate)(w526, w520) -> (w525:dbl[])
                  n326 = Build Array (concatenate)(w551, w545) -> (w550:cdb[])
                  n327 = local write "Reference Current (A)"(w550) -> ()
                  n328 = local write "Theta Device"(w525) -> ()
                }
                frame #2 {
                  # "Plot"
                  n329 = local read "Reference Current (A)"() -> (w574:dbl[])
                  n330 = local read "Device Current (A)"() -> (w575:dbl[])
                  n331 = local read "DC current (A)"() -> (w578:dbl[])
                  n332 = local read "Applied Biases (V)"() -> (w571:dbl[])
                  n333 = Divide(x=w575, y=w574) -> (x/y=w573:dbl[])
                  n334 = Divide(x=w573, y="Calibration Value") -> (x/y=w569:dbl[])
                  n335 = Bundle("Applied Biases (V)"=w571, "DC current (A)"=w578) -> (→"Device DC current":T9)  [unwired: 1 in]
                  n336 = Bundle("Applied Biases (V)"=w571, w569) -> (→"EQE(V)":cluster{"Applied Biases (V)":dbl[], dbl[]})  [unwired: 1 in]
                  n337 = Bundle("Applied Biases (V)"=w571, "Device Current (A)"=w575) -> (→"Device Lockin Current":T10)  [unwired: 1 in]
                  n338 = Bundle("Applied Biases (V)"=w571, "Reference Current (A)"=w574) -> (→"Reference Lockin Current":T11)  [unwired: 1 in]
                }
              }
              n339 = Greater Or Equal?(x=w505, y=w507) -> (x >= y?=w509:bool)
              n340 = Or(x=w509, y=w504) -> (x .or. y?=w508:bool)
            }
          }
          frame #2 {
            n341 = case shown="\"Scan\"" w584 {
              tunnel: w582 -> [w597 w635]
              tunnel: w583 -> [_ w632]
              frame "Calibrate", Default {
                w602 = 0
                # "Measure Currents on two lockins"
                # "Linear Interpolation of \ncalibration or\nphotodetector response"
                n342 = local read "Reference Current (A)"() -> (w600:dbl[])
                n343 = local read "Device Current (A)"() -> (w601:dbl[])
                n344 = Index Array(array=w601, index=w602) -> (element=w598:dbl)
                "Calib Photodet Current" <- w598
                n345 = Index Array(array=w600, index=w602) -> (element=w599:dbl)
                "Calib Ref Current" <- w599
                n346 = Unbundle(w597) -> ("Wavelength (nm)"=w603:sgl)  [unwired: 1 out]
                n347 = call-poly <vilib>:"Read From Spreadsheet File.vi"("file path (dialog if empty)"="Load Calibration Reference file") -> ("all rows"=w615:dbl[][])  [unwired: 6 in, 4 out]
                n348 = Divide(x=w598, y=w599) -> (x/y=w605:dbl)
                n349 = Index Array(array=w615, index (col)=0) -> (element=w609:dbl[])  [unwired: 1 in]
                n350 = Index Array(array=w615, index (col)=1) -> (element=w610:dbl[])  [unwired: 1 in]
                n351 = Build Array(w603) -> (w608:sgl[])
                n352 = call <vilib>:"Interpolate 1D.vi"("method"=1, "X is monotonic"=TRUE, "xi"=w608, "X"=w609, "Y"=w610) -> ("yi"=w607:dbl[])  [unwired: 4 in, 2 out]
                n353 = Index Array(array=w607, index=0) -> (element=w604:dbl)
                "Calib detector EQE" <- w604
                n354 = Divide(x=w605, y=w604) -> (x/y=w596:dbl)
                n355 = Absolute Value(x=w596) -> (abs(x)=w595:dbl)
                n356 = local write "Calibration Value"(w595) -> ()
              }
              frame "Scan" {
                w638 = TRUE
                w618 = "%g"
                # "Save Data"
                n357 = local read "Calib Photodet Current"() -> (w648:dbl)
                n358 = local read "Calib detector EQE"() -> (w649:dbl)
                n359 = Unbundle(w632) -> ("Wait (ms)"=w631:dbl, "Integration (ms)"=w630:u32)  [unwired: 3 out]
                n360 = local read "Calib Ref Current"() -> (w647:dbl)
                n361 = Unbundle(w635) -> ("Wavelength (nm)"=w634:sgl)  [unwired: 1 out]
                n362 = local read "Calibration Value"() -> (w646:dbl)
                n363 = Format Value(format string=w618, value (0)=w634) -> (output string=w633:string)  [unwired: 1 in]
                n364 = Format Value(format string=w618, value (0)=w649) -> (output string=w645:string)  [unwired: 1 in]
                n365 = Format Value(format string=w618, value (0)=w648) -> (output string=w644:string)  [unwired: 1 in]
                n366 = Format Value(format string=w618, value (0)=w647) -> (output string=w643:string)  [unwired: 1 in]
                n367 = Format Value(format string=w618, value (0)=w646) -> (output string=w642:string)  [unwired: 1 in]
                n368 = Format Value(format string=w618, value (0)=w631) -> (output string=w629:string)  [unwired: 1 in]
                n369 = Format Value(format string=w618, value (0)=w630) -> (output string=w628:string)  [unwired: 1 in]
                n370 = Build Array("Wavelength (nm)", "Calib detector EQE", "Calib Photodet Current (A)", "Calib Ref Current (A)", "Calibration value", "Wait time (ms)", "Integration time (ms)") -> (w651:string[])
                n371 = Build Array(w633, w645, w644, w643, w642, w629, w628) -> (w641:string[])
                n372 = Build Array("") -> (w623:string[])
                n373 = Build Array("Bias (V)", "EQE", "Device Current (A)", "Ref Current (A)", "DC device current (A)", "Theta of device (degrees)") -> (w624:string[])
                n374 = local read "DC current (A)"() -> (w616:dbl[])
                n375 = local read "Reference Current (A)"() -> (w664:dbl[])
                n376 = local read "Device Current (A)"() -> (w665:dbl[])
                n377 = Build Array(w651, w641, w623, w624) -> (w650:string[][])
                n378 = local read "Calibration Value"() -> (w658:dbl)
                n379 = local read "Applied Biases (V)"() -> (w617:dbl[])
                n380 = case shown="False" "Skip reset after\nmeasurement" {
                  tunnel: w650 -> [w669 _]
                  tunnel: [w668 w670] -> w640
                  tunnel: "Save File (Prompt if blank)" -> [w667 w670]
                  frame False {
                    n381 = call-poly <vilib>:"Write To Spreadsheet File.vi"("append to file? (new file:F)"=TRUE, "2D data"=w669, "file path (dialog if empty)"=w667) -> ("new file path (Not A Path if cancelled)"=w668:path)  [unwired: 5 in]
                  }
                  frame True {
                  }
                }
                n382 = Divide(x=w665, y=w664) -> (x/y=w657:dbl[])
                n383 = Divide(x=w657, y=w658) -> (x/y=w656:dbl[])
                n384 = local read "Theta Device"() -> (w620:dbl[])
                n385 = Build Array(w617, w656, w665, w664, w616, w620) -> (w637:dbl[][])
                n386 = call-poly <vilib>:"Write To Spreadsheet File.vi"("transpose? (no:F)"=w638, "format (%.3f)"="%g", "append to file? (new file:F)"=w638, "2D data"=w637, "file path (dialog if empty)"=w640) -> ()  [unwired: 3 in, 1 out]
              }
            }
            n387 = local read "Skip reset after\nmeasurement"() -> (w581:bool)
            n388 = case shown="False" w581 {
              frame False {
                # "Turn off Keithley output"
                n389 = call "Mono (YJ) - JPJ.vi"("Go to Wavelength"=0) -> ("Current Wavelength"=w585:dbl)  [unwired: 3 in, 2 out]
                n390 = local write "Current Wavelength"(w585) -> ()
                n391 = local read "Bias Parameters"() -> (w588:T5)
                n392 = Unbundle(w588) -> ("VISA resource name"=w587:refnum<visa-resource-name>)  [unwired: 4 out]
                n393 = call "Configure Output.vi"("VISA resource name"=w587) -> ("VISA resource name out"=w589:refnum<visa-resource-name>)  [unwired: 9 in, 1 out]
                n394 = call "Enable Output.vi"("Enable Output (T: Enable)"=FALSE, "VISA resource name"=w589) -> ("error out"=w591:errorcluster, "VISA resource name out"=w592:refnum<visa-resource-name>)  [unwired: 8 in]
                n395 = call "Close.vi"("error in (no error)"=w591, "VISA resource name"=w592) -> ("error out"=w593:errorcluster)  [unwired: 9 in]
                n396 = call <vilib>:"General Error Handler.vi"("error in (no error)"=w593) -> ()  [unwired: 10 in, 5 out]
              }
              frame True {
              }
            }
          }
        }
      }
    }
    "Gain (ohms, ref)" <- 1000 ("I-V resistance (ohms)")
    "Gain (ohms, device)" <- 1000 ("I-V resistance (ohms)")
  }
